vi "Create_Trajectory_Using_TrajectoryLibrary_NAT.vi"() -> ()   [LabVIEW 2019]
doc: "This utility creates trajectories based on the robot configuration, constraints and defined waypoints."
uses:
  <vilib>/Rock Robotics/WPI/ThirdParty/JAS_Junk/TrajLib/Trajectory_Library.lvlib
  <vilib>/Rock Robotics/WPI/ThirdParty/JAS_Junk/TrajLib/TypeDef/DISPLAY_WEIGHTED_WAYPOINT.ctl
  <vilib>/Rock Robotics/WPI/ThirdParty/JAS_Junk/TrajLib/TypeDef/TRAJECTORY.ctl
  <vilib>/Rock Robotics/WPI/ThirdParty/JAS_Junk/TrajLib/TypeDef/TRAJ_STATE.ctl
  <vilib>/Rock Robotics/WPI/ThirdParty/JAS_Junk/TrajLib/TypeDef/POSE2D.ctl
  <vilib>/Rock Robotics/WPI/ThirdParty/JAS_Junk/TrajLib/TypeDef/ROTATION2D.ctl
  <vilib>/Rock Robotics/WPI/ThirdParty/JAS_Junk/TrajLib/TypeDef/TRANSLATION2D.ctl
  CreateTrajectoryTypeDef/TrajCreateConfig_V3.ctl
  CreateTrajectoryENUM/TrajCreateUnitsENUM.ctl
  <vilib>/Rock Robotics/WPI/ThirdParty/JAS_Junk/TrajLib/TypeDef/TRAJ_CONSTRAINT_MECA_DRIVE_KINEMATICS.ctl
  <vilib>/Rock Robotics/WPI/ThirdParty/JAS_Junk/TrajLib/TypeDef/MECA_DRIVE_KINEMATICS.ctl
  <vilib>/Analysis/Matrix/Datatypes/RealMatrix.ctl
  <vilib>/Analysis/Matrix/NI_Matrix.lvlib
  <vilib>/Rock Robotics/WPI/ThirdParty/JAS_Junk/TrajLib/TypeDef/TRAJ_CONSTRAINT_DIIF_DRIVE_VOLTAGE.ctl
  <vilib>/Rock Robotics/WPI/ThirdParty/JAS_Junk/TrajLib/TypeDef/SIMPLE_MOTOR_FF.ctl
  <vilib>/Rock Robotics/WPI/ThirdParty/JAS_Junk/TrajLib/TypeDef/DIFF_DRIVE_KINEMATICS.ctl
  <vilib>/Rock Robotics/WPI/ThirdParty/JAS_Junk/TrajLib/TypeDef/TRAJ_CONSTRAINT_SWERVE_DRIVE_KINEMATICS.ctl
  <vilib>/Rock Robotics/WPI/ThirdParty/JAS_Junk/TrajLib/TypeDef/SWERVE_DRIVE_KINEMATICS.ctl
  <vilib>/Rock Robotics/WPI/ThirdParty/JAS_Junk/TrajLib/TypeDef/TRAJ_CONSTRAINT_CENTRIPETAL_ACCEL.ctl
  <vilib>/Utility/miscctls.llb/LVCursorListTypeDef.ctl
  <vilib>/Utility/xml.llb/Write to XML File(string).vi
  <vilib>/Utility/xml.llb/Read From XML File(string).vi
  <vilib>/Utility/inputDevices.llb/mouseAcquire.vi
  <vilib>/Rock Robotics/WPI/ThirdParty/JAS_Junk/TrajLib/TypeDef/SWERVE_DRIVE_MODULE_STATE.ctl
panel:
  out "CursIdx":i32
  out "Cursor Update Mode":i32=1
  out "Angle":dbl
  out "Scrolling":i32
  out "Index":i32
  in  "End Program":bool
  in  "Tab Control":T1(tab)
  out "Config File Read\nWithout Error":bool
  out "Config File  Read Error":errorcluster
  out "Read Config File Comment":string
  in  "Read Config File Name":path
  in  "ReadConfigFile":bool
  in  "Field Selector":string(combo)="2018 Power Up"
  in  "Units Selector":T2
  in  "MaxVelocity":dbl=50.0 format="%17.1f"
  in  "MaxAcceleration":dbl=40.0 format="%17.1f"
  out "MaxVelocity M/S":dbl=2.0 format="%17.4f"
  out "MaxAcceleration M/S^2":dbl=1.3 format="%17.4f"
  in  "Right Rear":T3={"X"=-0.5, "Y"=0.5} {"Y" format="%14.3f"; "X" format="%14.3f"}
  in  "Left Rear":T3={"X"=-0.5, "Y"=-0.5} {"Y" format="%14.3f"; "X" format="%14.3f"}
  in  "Right Front":T3={"X"=0.5, "Y"=0.5} {"Y" format="%14.3f"; "X" format="%14.3f"}
  in  "Left Front":T3={"X"=0.5, "Y"=-0.5} {"Y" format="%14.3f"; "X" format="%14.3f"}
  in  "Use Centripetal\nAcceleration\nConstaint":bool=TRUE
  out "Max Cent Accel M/S^2":dbl=1.0 format="%20.4f"
  in  "Max Cent Accel":dbl=20.0 format="%20.1f"
  in  "Use Diff Drive\nKinematic\nConstraint":bool=TRUE
  out "Wheelbase Width M":dbl=0.66 format="%20.4f"
  in  "Wheelbase Width":dbl=20.866 format="%20.1f"
  in  "Max Voltage":dbl=12.0 format="%20.4f"
  in  "SIMPLE_MOTOR_FF":T4={"Ks"=0.9, "Kv"=0.22199, "Ka"=0.04876, "KnInv"=0.0} {"KnInv" format="%13.4f"; "Ka" format="%13.4f"; "Kv" format="%13.4f"; "Ks" format="%13.4f"}
  in  "Use Diff Drive\nVoltage\nConstraint":bool=TRUE
  in  "Wheels":T3[](array[typedef])=[{"X"=0.5, "Y"=-0.5}, {"X"=0.5, "Y"=0.5}, {"X"=-0.5, "Y"=0.5}, {"X"=-0.5, "Y"=-0.5}] {"Y" format="%14.3f"; "X" format="%14.3f"}
  in  "Use Swerve Drive\nKinematics\nConstraint":bool
  in  "Use Mecanum \nDrive Kinematics\nConstraint":bool
  out "Left Front M":T3 {"Y" format="%14.3f"; "X" format="%14.3f"}
  out "Right Front M":T3 {"Y" format="%14.3f"; "X" format="%14.3f"}
  out "Left Rear M":T3 {"Y" format="%14.3f"; "X" format="%14.3f"}
  out "Right Rear M":T3 {"Y" format="%14.3f"; "X" format="%14.3f"}
  out "SIMPLE_MOTOR_FF M":T4 {"KnInv" format="%13.4f"; "Ka" format="%13.4f"; "Kv" format="%13.4f"; "Ks" format="%13.4f"}
  out "Wheels M":T3[](array[typedef]) {"Y" format="%14.3f"; "X" format="%14.3f"}
  in  "Remove Cursor":bool
  in  "Add Cursor":bool
  in  "Spline Type":enum32{"Radio Selection 1", "Radio Selection 2"}(radio)
  in  "Reverse":bool
  in  "UseWeights":bool
  in  "Calculate\nTrajectory":bool
  out "Trajectory\nCompleted\nError Free":bool
  out "Trajectory calculation error":errorcluster
  out "Position":cluster{dbl[], dbl[]}[](graph)
  out "Field Display":T5(plugin-control)
  in  "WayPoints":T6[](array[typedef])=[{"X"=15.0, "Y"=105.0, "ANGLE"=-45.0, "WEIGHT"=12.0}, {"X"=105.0, "Y"=65.0, "ANGLE"=0.0, "WEIGHT"=12.0}, {"X"=210.0, "Y"=106.0, "ANGLE"=45.0, "WEIGHT"=12.0}, {"X"=350.0, "Y"=105.0, "ANGLE"=-45.0, "WEIGHT"=12.0}] {"WEIGHT" format="%13.3f"; "ANGLE" format="%13.3f"; "Y" format="%13.3f"; "X" format="%13.3f"}
  out "Trajectory Data":cluster{dbl[], dbl[]}[](graph)
  out "differential \ndrive \nmax speed":dbl format="%15.1f"
  out "Traj States\nSize":i32
  out "Trajectory States":T7[](array[typedef]) {"POSE"."ROTATION"."SIN" format="%13.4f"; "POSE"."ROTATION"."COS" format="%13.4f"; "POSE"."ROTATION"."VALUE" format="%13.4f"; "POSE"."TRANSLATION"."Y" format="%14.3f"; "POSE"."TRANSLATION"."X" format="%14.3f"}
  in  "Trajectory JSON File Name":path
  out "JSON File Saved\nWithout Error":bool
  out "Write CSV File Error":errorcluster
  in  "PathWeaver Length Units":T10(radio)
  in  "WriteJSONFile":bool
  out "CSV File Saved\nWithout Error":bool
  in  "Trajectory Type":enum32{"Radio Selection 1", "Radio Selection 2"}(radio)
  out "Write Trajectory\nFile Error":errorcluster
  in  "Trajectory File Comment":string
  in  "Trajectory CSV File Name":path
  in  "WriteTrajFile":bool
  out "Config File Saved\nWithout Error":bool
  out "Write Config FIle Error":errorcluster
  in  "Write Config File Comment":string
  in  "Write Config File Name":path
  in  "WriteConfigFile":bool
  # "Create Trajectory  (Use LabVIEW trajectory library)"
  # "Instructions:  \n----------------\n\nThis utility will create a trajectory, show the data on the various tabs, and optionally write a \"field absolute\" or \"robot relative\" trajectory to a file. \nTo use this utility:\n\n1) Read all of these instructions!\n2) Define the robot's physical data on the \"Robot Data\" tab.  \n3) Define the robot's movement constraints on the \"Constraints\" page.  \n4) Define the trajectory on the \"Define/Create Trajectory\" tab.  These are the beginning and ending positions/headings, and internal positions/headings.  \n    Cubic splines only use the first and last \"angle\".  The other internal \"angles\" are calculated.  Quintic splines use all the defined angles.\n5) Press the \"Calculate Trajectory\".  If a good trajectory was calculated it will be displayed.  If no errors are generated the Trajectory Complete\n    light will be on.  Errors will be displayed in the error indicator.  The path can be recalculated many times before performing any other action.\n\nAfter a Trajectory has been calculated, the \"trajectory can be written to a file.  The absolute path is converted to a robot relative trajectory.  To do this:\n1) Enter a comment to be included in the file.  Anything can be entered.\n2) Select the file name.\n3) Press \"Create Trajectory File\"  If an error occurs it will be displayed in the File Creation Error indicator.\n\nNotes:\n--------\n- All the robot parameters, path, and field dimensions are in UNITS, and DEGREES.  Select UNITS from the \"Robot Data\" page.  The resulting  \n  trajectory is converted to METERS, and RADIANS to match the rest of this library!\n- The trajectory library is the same as the WPILIB spline and trajectory library for Java and C++.\n- 2019 playing field size - width: 26 ft 11.25 In = 323.25 in , length: 52 ft 5.25 in = 629.25 in  (I didn't verify this for the 2020 version.)"
  # "Read Trajectory Waypoints and Configuration from File"
  # "ROBOT DATA"
  # "UNITS/SEC"
  # "Meters/SEC"
  # "UNITS/SEC^2"
  # "Meters/SEC^2"
  # "Simulated robot max speed is: 68.266 Inches/Second"
  # "UTILITY CONFIGURATION"
  # "Diff Kinematics Constraint"
  # "Centripetal Accel Constraint"
  # "Diff Voltage Constraint"
  # "UNITS"
  # "UNITS/SEC^2"
  # "VOLTS"
  # "METERS"
  # "METERS/SEC^2"
  # "Distance is:\nUNITS"
  # "Simulated robot wheelbase is 20.87 in"
  # "Ks = Volts\nKv = VoltSec/Meter\nKa = Volt(Sec^2)/Meter"
  # "Swerve Kinematics Constraint"
  # "Mechanum Kinematics Constraint"
  # "Values\nare \nUNITS"
  # "Values\nare \nUNITS"
  # "TRAJECTORY DEFINITION"
  # "To delete array elements or the entire array, right click on the array or element, select Data Operations, then select the action to be performed."
  # "UNITS, UNITS, DEGREES, SCALAR"
  # "INCHES/SEC"
  # "Write Trajectory to File   -   CSV, and / or JSON"
  # "Write Trajectory Waypoints and Configuration to File"
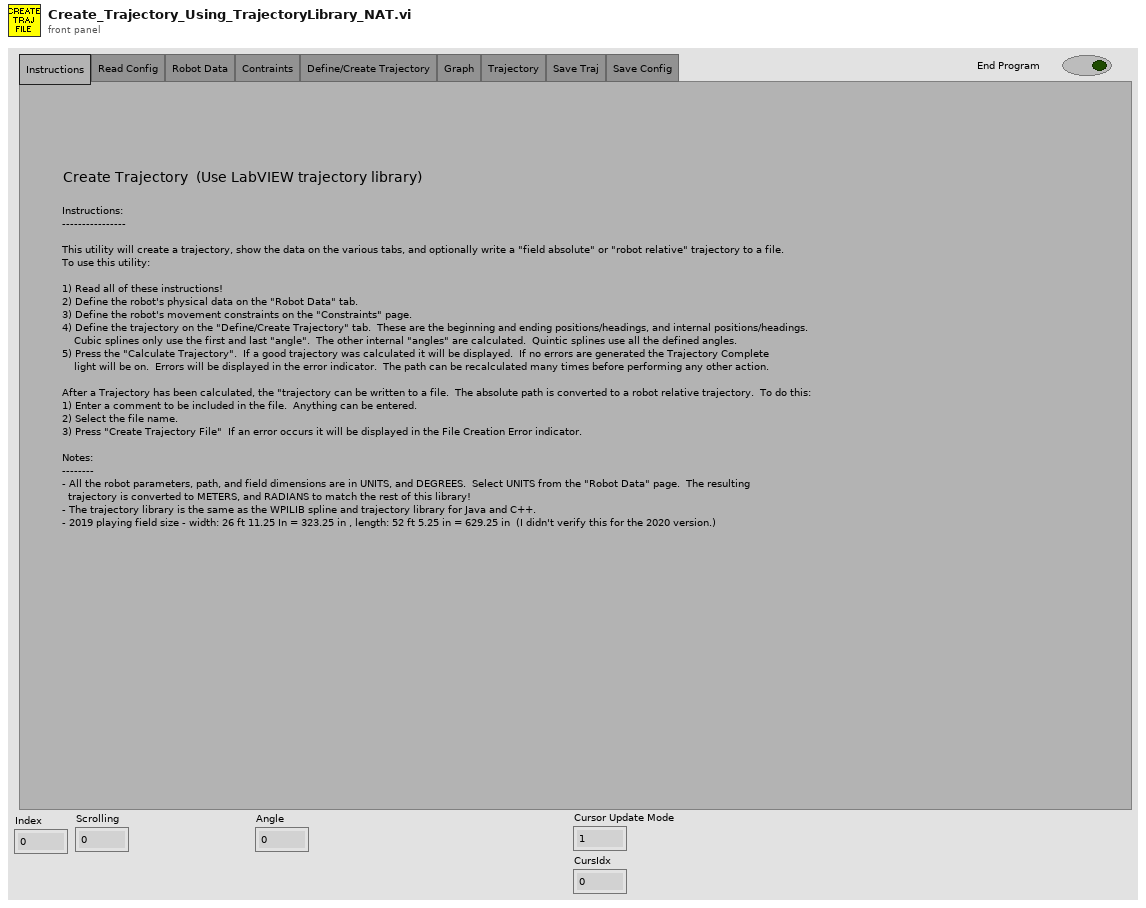
[diagram p1: front panel]
types:
  T1 = enum32{"Instructions", "Read Config", "Robot Data", "Contraints", "Define/Create Trajectory", "Graph", "Trajectory", "Save Traj", "Save Config"}
  T2 = typedef "TrajCreateUnitsENUM.ctl" = enum16{"Inches", "Feet", "Centimeters", "Meters"}
  T3 = typedef "Trajectory_Library.lvlib/TRANSLATION2D.ctl" = cluster{"X":dbl, "Y":dbl}
  T4 = typedef "Trajectory_Library.lvlib/SIMPLE_MOTOR_FF.ctl" = cluster{"Ks":dbl, "Kv":dbl, "Ka":dbl, "KnInv":dbl}
  T5 = typedef "IMAQ Image.ctl" = refnum<image>
  T6 = typedef "Trajectory_Library.lvlib/DISPLAY_WEIGHTED_WAYPOINT.ctl" = cluster{"X":dbl, "Y":dbl, "ANGLE":dbl, "WEIGHT":dbl}
  T7 = typedef "Trajectory_Library.lvlib/TRAJ_STATE.ctl" = cluster{"TimeSeconds":dbl, "Velocity":dbl, "Acceleration":dbl, "POSE":T8, "Curvature":dbl}
  T8 = typedef "Trajectory_Library.lvlib/POSE2D.ctl" = cluster{"TRANSLATION":T3, "ROTATION":T9}
  T9 = typedef "Trajectory_Library.lvlib/ROTATION2D.ctl" = cluster{"VALUE":dbl, "COS":dbl, "SIN":dbl}
  T10 = enum32{"Radio Selection 1", "Radio Selection 2", "Radio Selection 3", "Radio Selection 4", "Radio Selection 5"}
  T11 = typedef "LVCursorListTypeDef.ctl" = cluster{"Name":string, "Color":u32, "Style":u8, "Point Style":u8, "Name Visible":bool, "Allow Drag":bool, "Cursor Mode":u32, "Plot":i32, "Index":i32, "Position":cluster{"X":dbl, "Y":dbl}, "X Scale":u32, "Y Scale":u32, "Watch Plots":i32[], "Watch All Plots":bool, "Plot Area":i32, "Label Offset":cluster{"X":dbl, "Y":dbl}}[]
  T12 = typedef "Image Type" = u32
  T13 = typedef "Trajectory_Library.lvlib/TRAJECTORY.ctl" = cluster{"TotalTImeSecs":dbl, "States":T7[]}
  T14 = typedef "TrajCreateConfig_V3.ctl" = cluster{"Write Config File Name":path, "Write Config File Comment":string, "WayPoints":T6[], "TRAJECTORY_CONFIG":cluster{"MaxVelocity":dbl, "Max Acceleration":dbl, "StartVelocity":dbl, "End Velocity":dbl, "Reversed":bool, "DiffDrKineConstntDefined":bool, "CentAcellConstntDefined":bool, "DiffDrVoltConstntDefined":bool, "DIFF_DRIVE_KINE_CONSTRAINT":cluster{"Max Speed (M/S)":dbl, "DIFF_DRIVE_KINEMATICS":T15}, "CENTRIPETAL_ACCEL_CONSTRAINT":T16, "SwerveDrKineConstntDefined":bool, "SWERVE_DRIVE_KINE_CONSTRAINT":T17, "DIFF_DRIVE_VOLTAGE_CONSTRAINT":T21, "MECANUM_DRIVE_KINE_CONSTRAINT":T22, "MecanumDrKineConstntDefined":bool}, "IsCubic":bool, "Units Selector":T2, "UseWeights":bool}
  T15 = typedef "Trajectory_Library.lvlib/DIFF_DRIVE_KINEMATICS.ctl" = cluster{"TrackWidth_Meters":dbl}
  T16 = typedef "Trajectory_Library.lvlib/TRAJ_CONSTRAINT_CENTRIPETAL_ACCEL.ctl" = cluster{"Max Cent Accel":dbl}
  T17 = typedef "Trajectory_Library.lvlib/TRAJ_CONSTRAINT_SWERVE_DRIVE_KINEMATICS.ctl" = cluster{"Max Speed (M/S)":dbl, "SwerveKinematics":T18}
  T18 = typedef "Trajectory_Library.lvlib/SWERVE_DRIVE_KINEMATICS.ctl" = cluster{"NumModules":i32, "InverseKinematics":T19, "ForwardKinematics":T19, "Modules":T3[], "PrevCoR":T3, "SavedModuleStates":T20[]}
  T19 = typedef "NI_Matrix.lvlib/RealMatrix.ctl" = dbl[][]
  T20 = typedef "Trajectory_Library.lvlib/SWERVE_DRIVE_MODULE_STATE.ctl" = cluster{"Speed":dbl, "Angle":T9}
  T21 = typedef "Trajectory_Library.lvlib/TRAJ_CONSTRAINT_DIIF_DRIVE_VOLTAGE.ctl" = cluster{"Max Voltage":dbl, "DIFF_DRIVE_KINEMATICS":T15, "SIMPLE_MOTOR_FF":T4}
  T22 = typedef "Trajectory_Library.lvlib/TRAJ_CONSTRAINT_MECA_DRIVE_KINEMATICS.ctl" = cluster{"Max Speed (M/S)":dbl, "MECA_DRIVE_KINEMATICS":T23}
  T23 = typedef "Trajectory_Library.lvlib/MECA_DRIVE_KINEMATICS.ctl" = cluster{"FrontLeft":T3, "FrontRight":T3, "RearLeft":T3, "RearRight":T3, "InverseKinematics":T19, "ForwardKinematics":T19, "PrevCoR":T3}
  T24 = cluster{"Name":string, "Color":u32, "Style":u8, "Point Style":u8, "Name Visible":bool, "Allow Drag":bool, "Cursor Mode":u32, "Plot":i32, "Index":i32, "Position":cluster{"X":dbl, "Y":dbl}, "X Scale":u32, "Y Scale":u32, "Watch Plots":i32[], "Watch All Plots":bool, "Plot Area":i32, "Label Offset":cluster{"X":dbl, "Y":dbl}}
  T25 = enum8{"Enabled", "Disabled", "Disabled and Grayed Out"}
  T26 = cluster{"Horizontal":i32, "Vertical":i32, "Scrolling":i32}
  T27 = typedef "TrajectoryUtils_Field_Info.ctl" = cluster{"FIeld_File_Name":string, "Top_Left_X":i32, "Top_Left_Y":i32, "Bottom_Right_X":i32, "Bottom_Right_Y":i32, "Field_Size_X":dbl, "Field_Size_Y":dbl, "FIeld_Size_Units":string}
  T28 = typedef "TrajCreateConfig__V_Internal.ctl" = cluster{"Write Config File Name":path, "Write Config File Comment":string, "WayPoints":T6[], "TRAJECTORY_CONFIG":T29, "IsCubic":bool, "Units Selector":T2, "UseWeights":bool, "FieldName":string}
  T29 = typedef "Trajectory_Library.lvlib/TRAJ_CONFIG.ctl" = cluster{"MaxVelocity":dbl, "Max Acceleration":dbl, "StartVelocity":dbl, "End Velocity":dbl, "Reversed":bool, "Constraints":variant[]}
  T30 = typedef "Trajectory_Library.lvlib/TRAJ_CONSTRAINT_DIIF_DRIVE_KINEMATICS.ctl" = cluster{"Max Speed (M/S)":dbl, "DIFF_DRIVE_KINEMATICS":T15, "Max Accel (M/S2)":dbl}
  T31 = typedef "Trajectory_Library.lvlib/TRAJ_CONSTRAINT_DIIF_DRIVE_VOLTAGE.ctl" = cluster{"Max Voltage":dbl, "DIFF_DRIVE_KINEMATICS":T15, "SIMPLE_MOTOR_FF":T32}
  T32 = typedef "Trajectory_Library.lvlib/SIMPLE_MOTOR_FF.ctl" = cluster{"Ks":dbl, "Kv":dbl, "Ka":dbl}
  T33 = typedef "Trajectory_Library.lvlib/TRAJ_CONSTRAINT_SWERVE_DRIVE_KINEMATICS.ctl" = cluster{"Max Speed (M/S)":dbl, "SwerveKinematics":T34}
  T34 = typedef "Trajectory_Library.lvlib/SWERVE_DRIVE_KINEMATICS.ctl" = cluster{"NumModules":i32, "InverseKinematics":T19, "ForwardKinematics":T19, "Modules":T3[], "PrevCoR":T3}
  T35 = typedef "Trajectory_Library.lvlib/WEIGHTED_WAYPOINT.ctl" = cluster{"TRANSLATION":T3, "ROTATION":T9, "SCALAR":dbl}
  T36 = typedef "Trajectory_Library.lvlib/SPLINE_CTRL_VECTOR.ctl" = cluster{"Xs":dbl[], "Ys":dbl[]}
  T37 = typedef "Trajectory_Library.lvlib/CHASSIS_SPEEDS.ctl" = cluster{"vX":dbl, "vY":dbl, "vOmega":dbl}
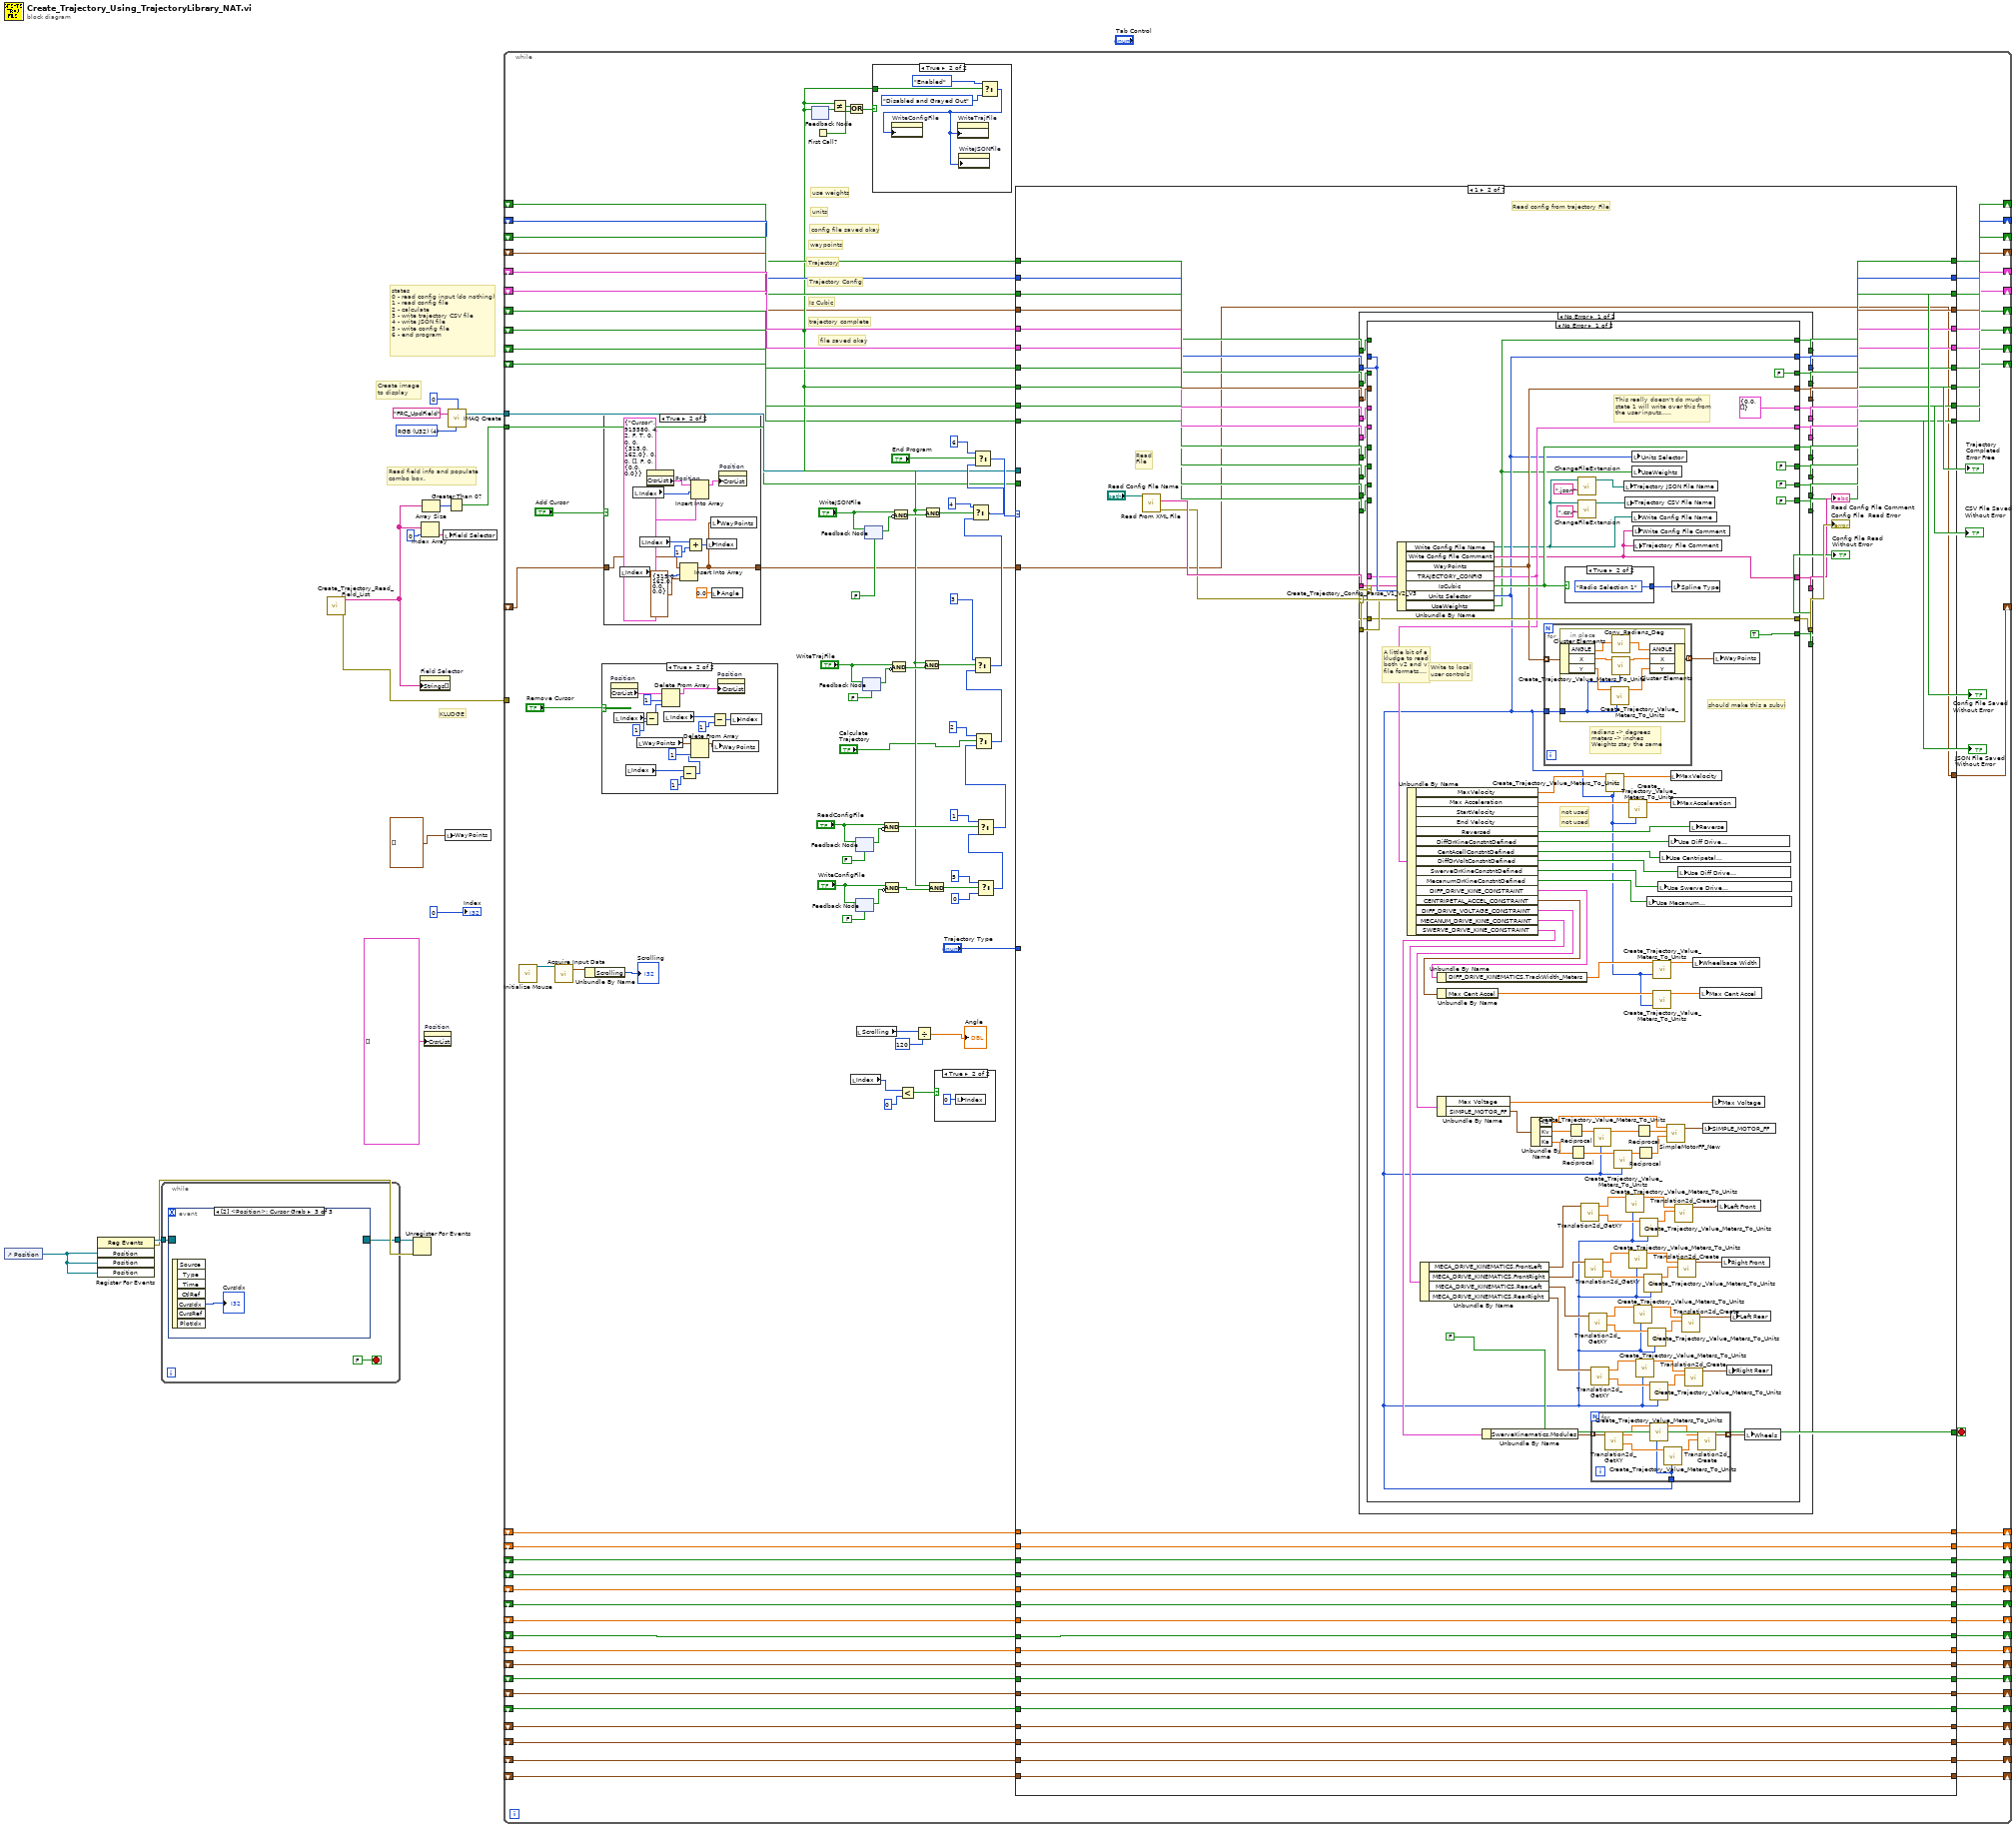
[diagram p0: block diagram]
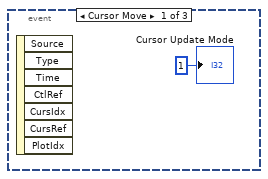
[diagram p2: hidden frame]
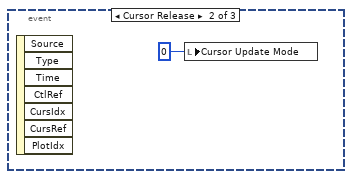
[diagram p3: hidden frame]
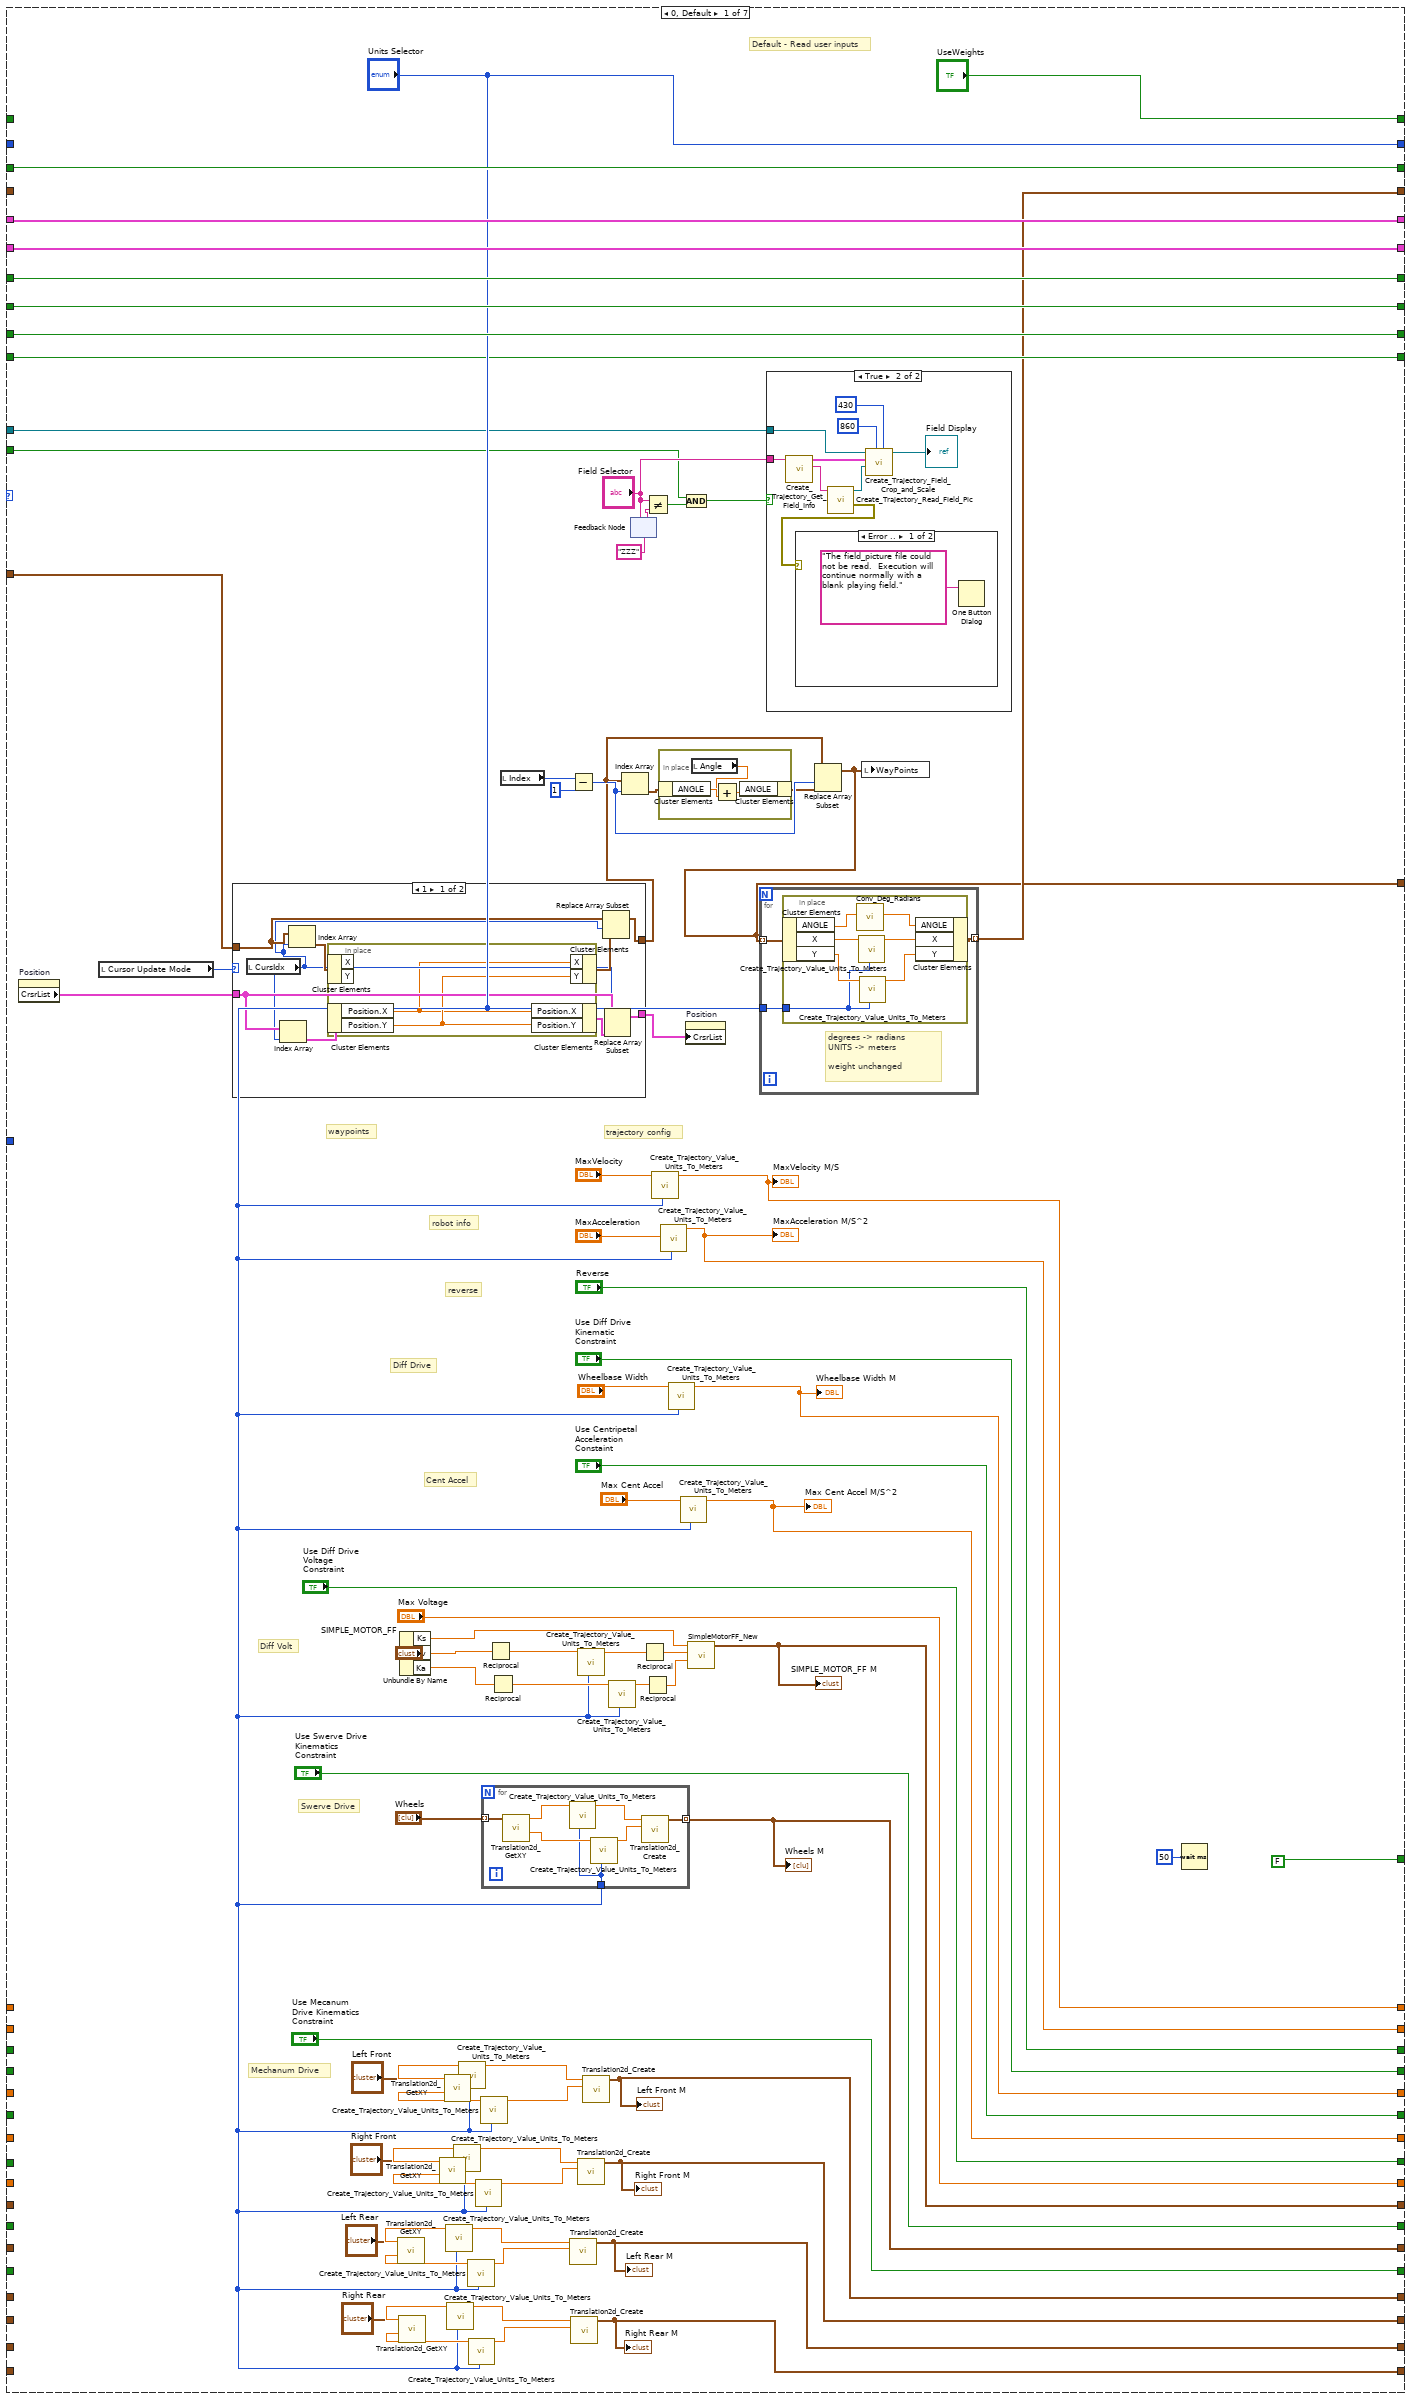
[diagram p4: hidden frame]
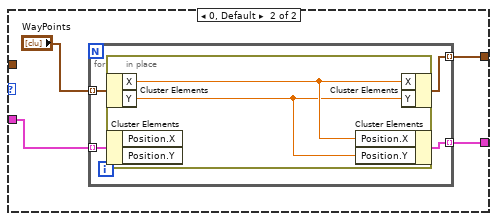
[diagram p5: hidden frame]
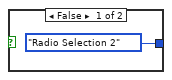
[diagram p8: hidden frame]
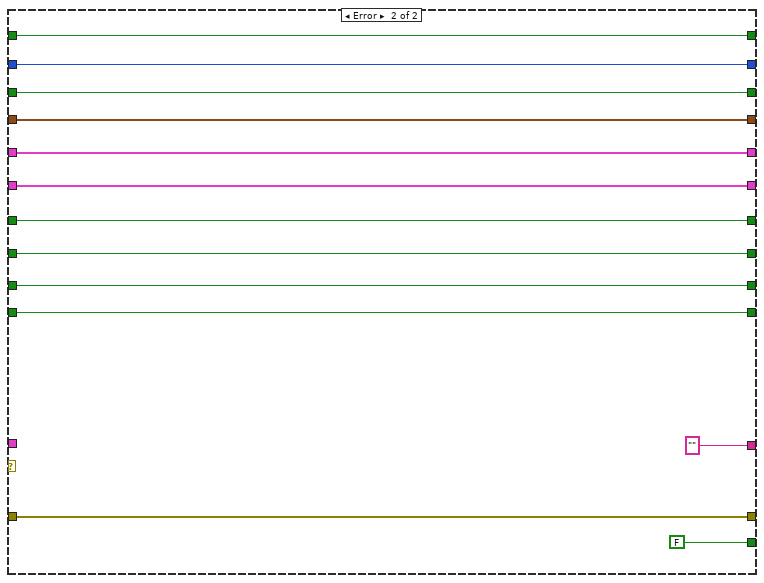
[diagram p9: hidden frame]
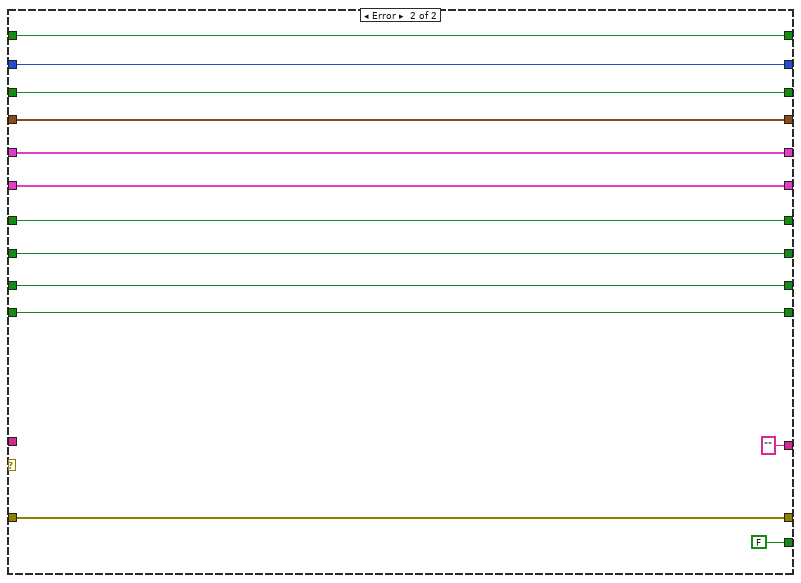
[diagram p10: hidden frame]
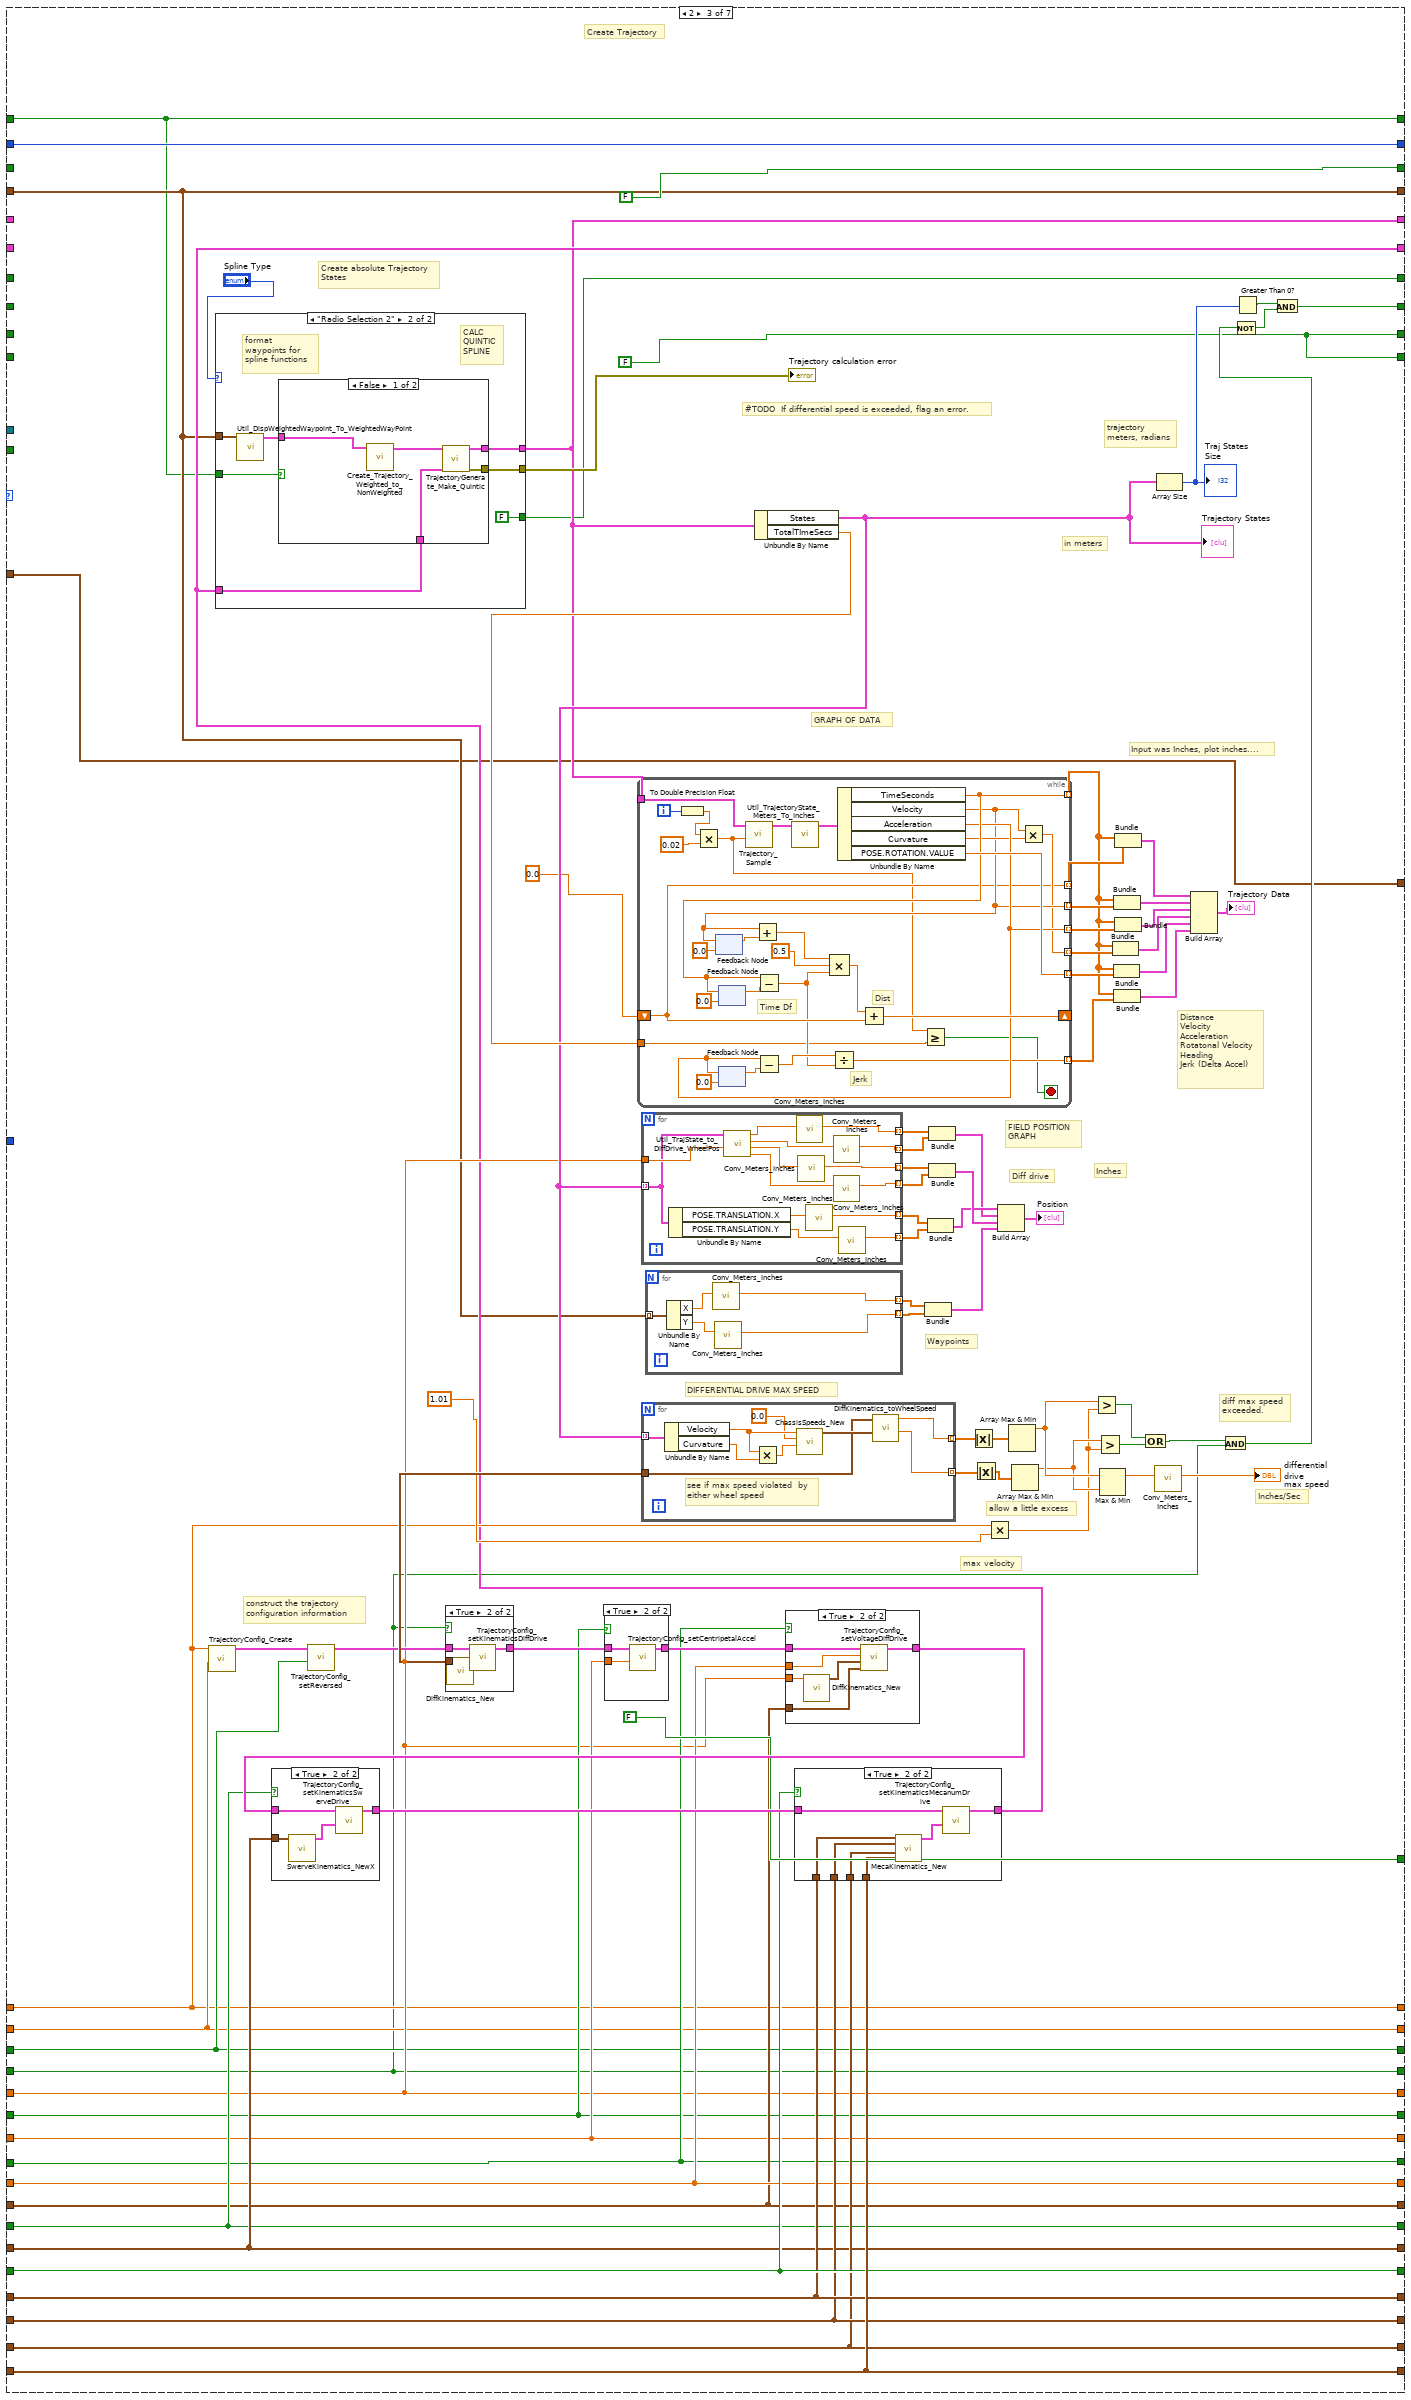
[diagram p11: hidden frame]
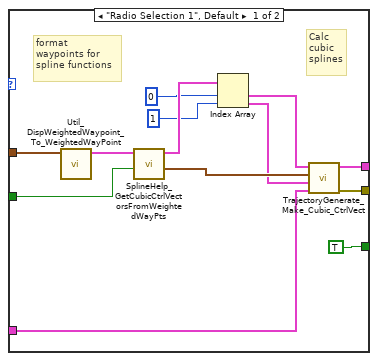
[diagram p13: hidden frame]
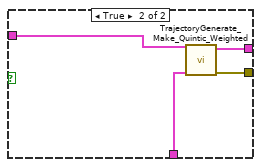
[diagram p14: hidden frame]
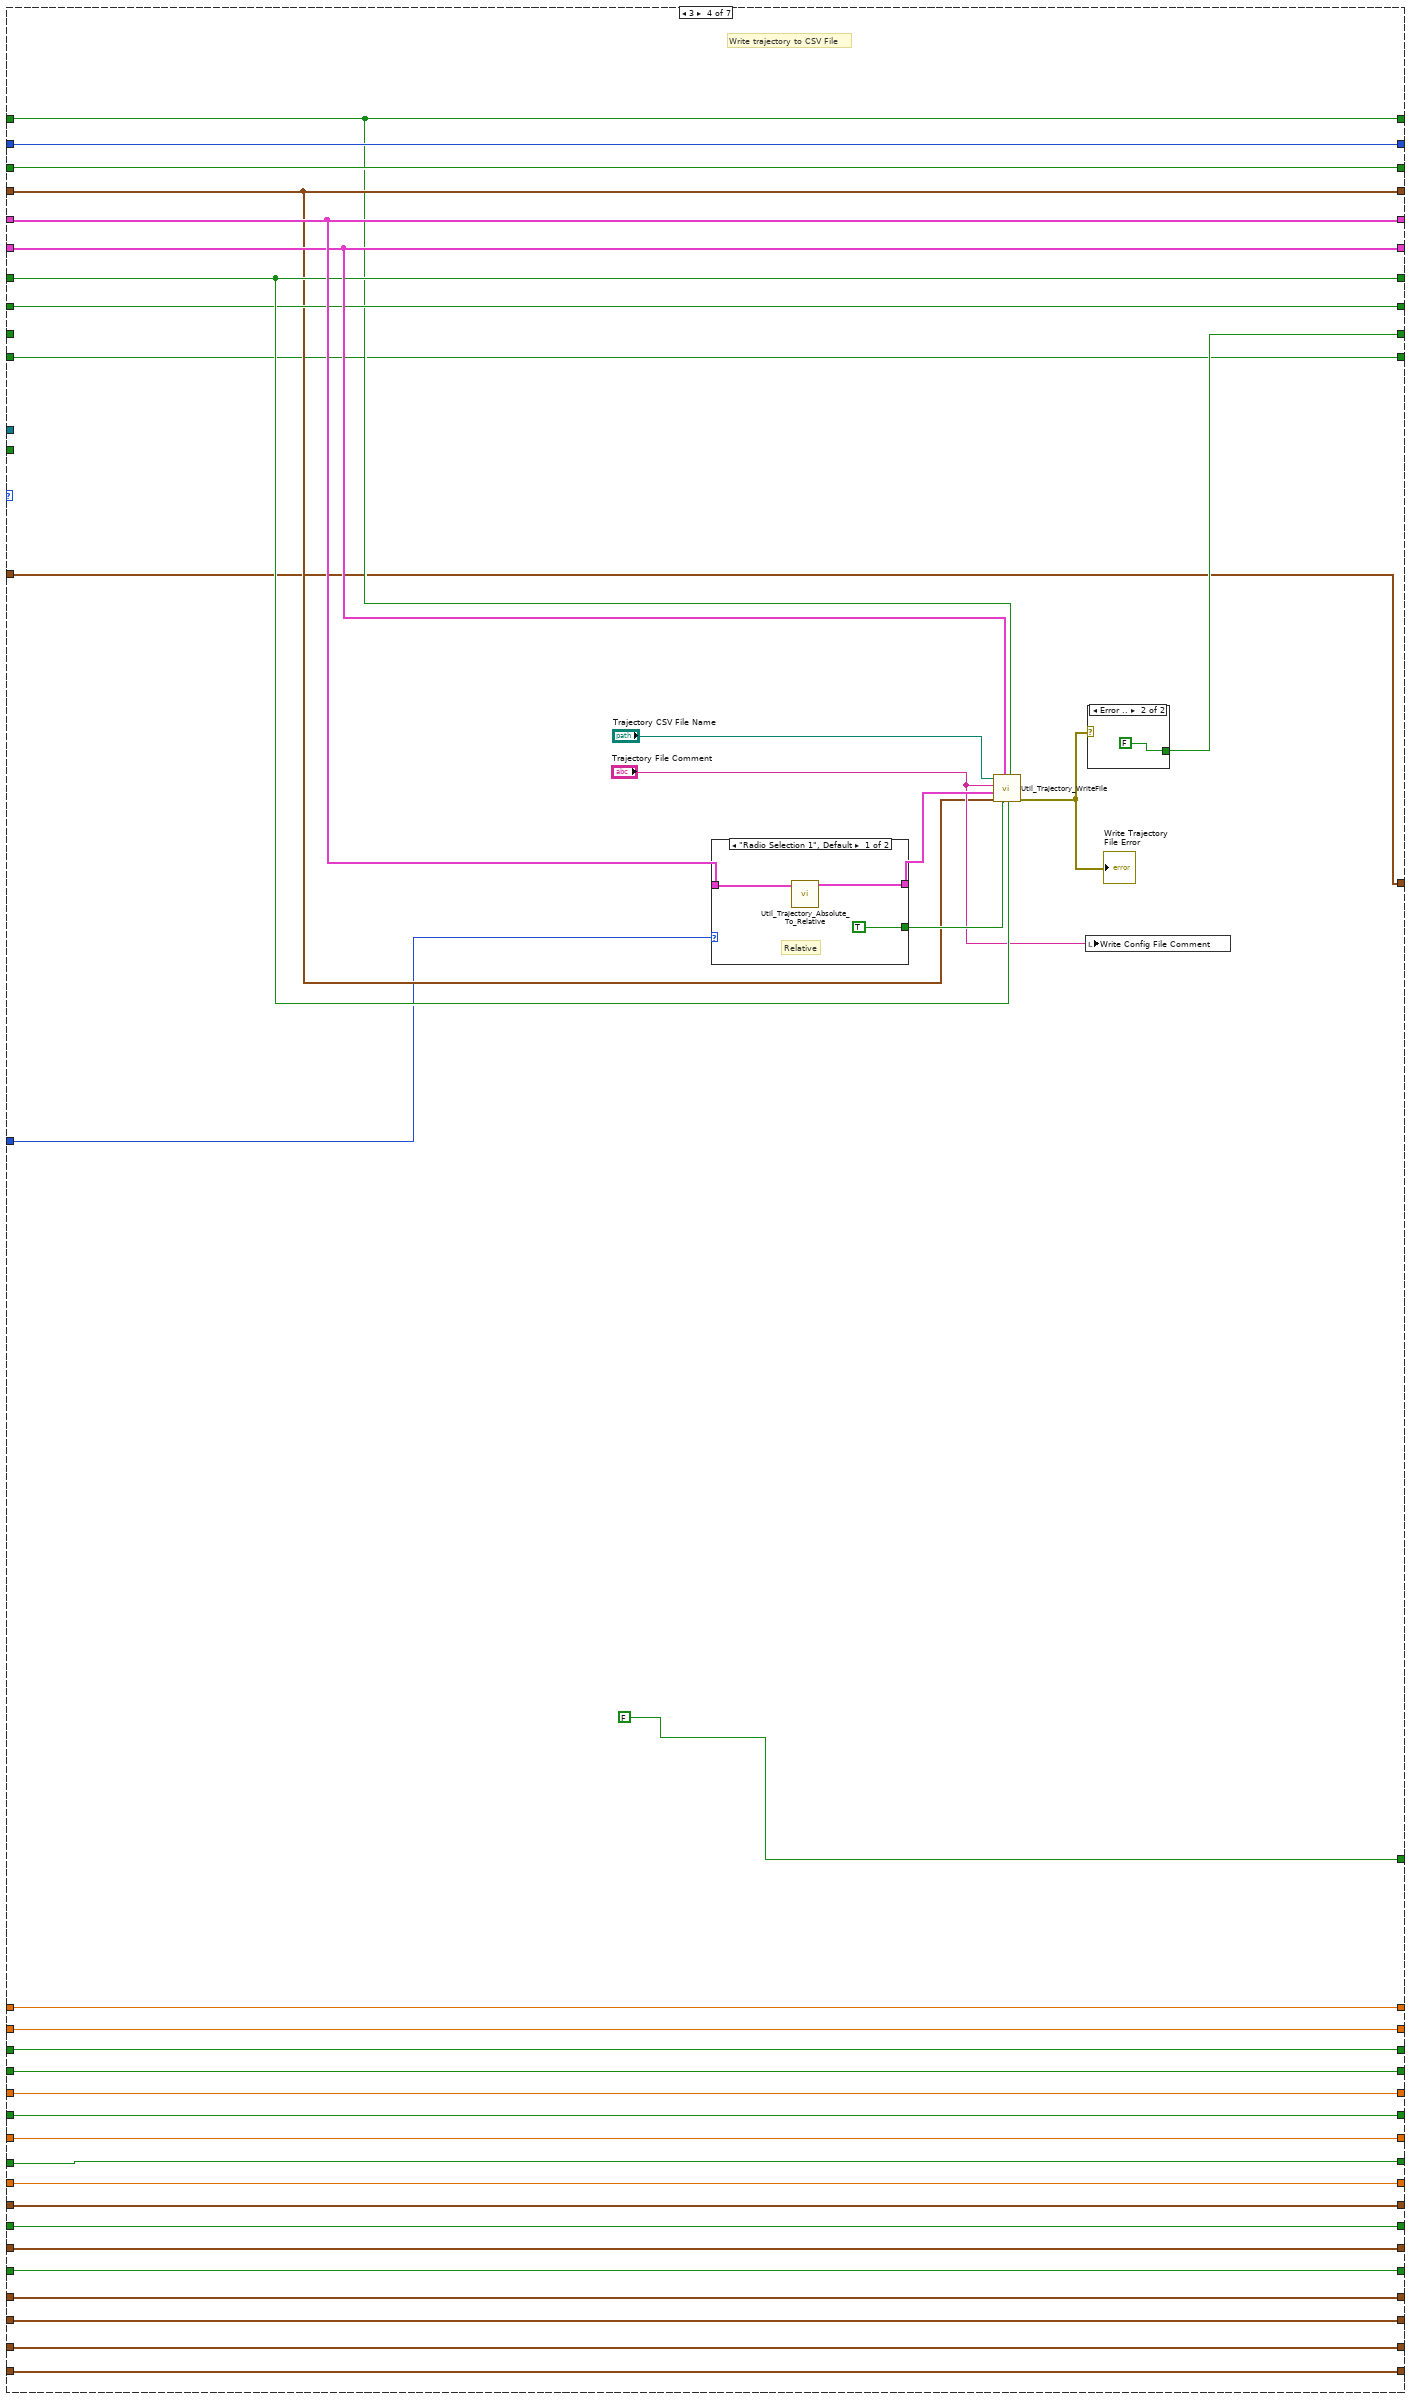
[diagram p19: hidden frame]
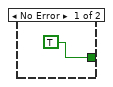
[diagram p20: hidden frame]
diagram:
  w12 = T12 4 items=["Grayscale (U8)", "Grayscale (I16)", "Grayscale (SGL)", "Complex (CSG)", "RGB (U32)", "HSL (U32)", "RGB (U64)", "Grayscale (U16)"] ("Image Type")
  # "Create image \nto display"
  # "KLUDGE"
  # "Read field info and populate\ncombo box."
  # "states\n0 - read config input (do nothing)\n1 - read config file\n2 - calculate\n3 - write trajectory CSV file\n4 - write JSON file\n5 - write config file\n6 - end program"
  n1 = control-ref of="Position"() -> (w4:refnum<vi>)
  n2 = register-events(w4, w4, w4) -> (reference out=w3:refnum<event-registration>, error out=w1:errorcluster)  [unwired: 2 in]
  n3 = while {
    tunnel: w3 -> [w20]
    tunnel: [w19] -> w2
    stop <- FALSE stop-if-true
    n4 = event shown="[2] <Position>: Cursor Grab" {
      selector: w20 -> [_ _ _]
      dyn-events: [_ _ _] -> w19
      timeout: _ -> [_ _ _]
      event Cursor Move {
        n5 = event-data() -> ()  [unwired: 1 in, 7 out]
        "Cursor Update Mode" <- 1
      }
      event Cursor Release {
        n6 = event-data() -> ()  [unwired: 1 in, 7 out]
        n7 = local write "Cursor Update Mode"(0 ("Wapoint Update Mode")) -> ()
      }
      event Cursor Grab {
        n8 = event-data() -> ("CursIdx"=→"CursIdx":i32)  [unwired: 1 in, 6 out]
      }
    }
  }
  n9 = call "Create_Trajectory_Read_Field_List.vi"() -> ("error out"=w15:errorcluster, "section names"=w10:string[])  [unwired: 10 in]
  n10 = Unregister For Events(event registration refnum=w2, error in=w1) -> ()  [unwired: 1 out]
  n11 = property on="Field Selector" class="CmbBox"("Strings[]"=w10) -> ()  [unwired: 2 in, 2 out]
  n12 = Index Array(array=w10, index=0) -> (element=w16:string)
  n13 = Array Size(array=w10) -> (size(s)=w9:i32)
  n14 = property on="Position" class="XYGraph (strict)"("CrsrList"=T11 [] ("Cursor List")) -> ()  [unwired: 2 in, 2 out]
  n15 = local write "Field Selector"(w16) -> ()
  n16 = local write "WayPoints"(T6[] [] ("WayPoints")) -> ()
  n17 = Greater Than 0?(x=w9) -> (x > 0?=w8:bool)
  n18 = call "IMAQ Create"("Border Size"=0, "Image Name"="FRC_UpdField", "Image Type"=w12) -> ("New Image"=w11:T5)  [unwired: 2 in, 1 out]
  n19 = while {
    shift-right: [w127] -> _
    shift-left: _ -> [w126]
    shift-right: [w125] -> _
    shift-left: _ -> [w124]
    shift-right: [w111] -> _
    shift-left: _ -> [w112]
    shift-right: [w113] -> _
    shift-left: _ -> [w29]
    shift-right: [w110] -> _
    shift-left: _ -> [w50]
    shift-right: [w106] -> _
    shift-left: _ -> [w107]
    shift-right: [w96] -> _
    shift-left: _ -> [w101]
    shift-right: [w105] -> _
    shift-left: _ -> [w100]
    shift-right: [w97] -> _
    shift-left: _ -> [w104]
    shift-right: [w98] -> _
    shift-left: _ -> [w103]
    shift-right: [w99] -> _
    shift-left: _ -> [w102]
    shift-right: [w95] -> _
    shift-left: _ -> [w93]
    shift-right: [w94] -> _
    shift-left: _ -> [w92]
    shift-right: [w89] -> _
    shift-left: _ -> [w90]
    shift-right: [w88] -> _
    shift-left: _ -> [w91]
    shift-right: [w86] -> _
    shift-left: _ -> [w87]
    shift-right: [w82] -> _
    shift-left: _ -> [w84]
    shift-right: [w83] -> _
    shift-left: _ -> [w85]
    shift-right: [w79] -> _
    shift-left: _ -> [w81]
    shift-right: [w78] -> _
    shift-left: _ -> [w80]
    shift-right: [w72] -> _
    shift-left: _ -> [w75]
    shift-right: [w73] -> _
    shift-left: _ -> [w76]
    shift-right: [w74] -> _
    shift-left: _ -> [w77]
    shift-right: [w60] -> _
    shift-left: _ -> [w59]
    shift-right: [w58] -> _
    shift-left: _ -> [w57]
    shift-right: [w56] -> _
    shift-left: _ -> [w55]
    shift-right: [w45] -> _
    shift-left: _ -> [w44]
    tunnel: w15 -> [_]
    tunnel: w11 -> [w42]
    tunnel: w8 -> [w41]
    shift-right: [w28] -> _
    shift-left: _ -> [w27]
    stop <- w108 stop-if-true
    # "use weights"
    # "units"
    # "config file saved okay"
    # "file saved okay"
    # "trajectory complete"
    # "Is Cubic"
    # "waypoints"
    # "Trajectory Config"
    # "Trajectory"
    n20 = call <vilib>:"Initialize Mouse.vi"() -> ("device ID"=w33:refnum<k1>)  [unwired: 10 in, 1 out]
    n21 = call-poly <vilib>:"Acquire Input Data.vi"("device ID"=w33) -> ("axis info"=w34:T26)  [unwired: 15 in, 3 out]
    n22 = Unbundle By Name(w34) -> ("Scrolling"=→"Scrolling":i32)
    n23 = case shown="True" "Remove Cursor" {
      frame False {
      }
      frame True {
        n24 = property on="Position" class="XYGraph (strict)"() -> ("CrsrList"=w922:T11)  [unwired: 2 in, 2 out]
        n25 = local read "Index"() -> (w913:i32)
        n26 = local read "Index"() -> (w908:i32)
        n27 = local read "WayPoints"() -> (w915:T6[])
        n28 = Subtract(x=w913, y=1) -> (x-y=w911:i32)
        n29 = Delete From Array(array=w922, length=1, index=w911) -> (array with subset deleted=w920:T11)  [unwired: 1 out]
        n30 = local read "Index"() -> (w919:i32)
        n31 = Subtract(x=w908, y=1) -> (x-y=w909:i32)
        n32 = Delete From Array(array=w915, length=1, index=w909) -> (array with subset deleted=w916:T6[])  [unwired: 1 out]
        n33 = Subtract(x=w919, y=1) -> (x-y=w917:i32)
        n34 = local write "WayPoints"(w916) -> ()
        n35 = property on="Position" class="XYGraph (strict)"("CrsrList"=w920) -> ()  [unwired: 2 in, 2 out]
        n36 = local write "Index"(w917) -> ()
      }
    }
    n37 = case shown="True" "Add Cursor" {
      tunnel: [w923 w925] -> w30
      tunnel: w27 -> [w923 w924]
      frame False {
      }
      frame True {
        n38 = local read "Index"() -> (w929:i32)
        n39 = local read "Index"() -> (w934:i32)
        n40 = local read "Index"() -> (w931:i32)
        n41 = property on="Position" class="XYGraph (strict)"() -> ("CrsrList"=w935:T11)  [unwired: 2 in, 2 out]
        n42 = Insert Into Array(array=w924, index=w929, new element=T6 {"X"=315.0, "Y"=162.0, "ANGLE"=0.0, "WEIGHT"=0.0} ("new element/subarray")) -> (w925:T6[])
        n43 = Add(x=w931, y=1) -> (x+y=w933:i32)
        n44 = Insert Into Array(array=w935, index=w934, new element=T24 {"Name"="Cursor", "Color"=915580, "Style"=4, "Point Style"=2, "Name Visible"=FALSE, "Allow Drag"=TRUE, "Cursor Mode"=0, "Plot"=0, "Index"=0, "Position"={"X"=315.0, "Y"=162.0}, "X Scale"=0, "Y Scale"=0, "Watch Plots"=[], "Watch All Plots"=FALSE, "Plot Area"=0, "Label Offset"={"X"=0.0, "Y"=0.0}} ("new element/subarray")) -> (w930:T11)
        n45 = local write "Index"(w933) -> ()
        n46 = local write "WayPoints"(w925) -> ()
        n47 = local write "Angle"(0.0 ("Angle")) -> ()
        n48 = property on="Position" class="XYGraph (strict)"("CrsrList"=w930) -> ()  [unwired: 2 in, 2 out]
      }
    }
    n49 = feedback #1() -> (w64:bool)  [unwired: 1 in]
    n50 = feedback-in #1(w50) -> ()
    n51 = First Call?() -> (First Call?: T/F=w62:bool)
    n52 = Not Equal?(x=w50, y=w64) -> (x != y?=w63:bool)
    n53 = Or(x=w63, y=w62) -> (x .or. y?=w61:bool)
    n54 = local read "Index"() -> (w40:i32)
    n55 = feedback #2(FALSE ("CreateCmdList")) -> (w130:bool)
    n56 = feedback-in #2("ReadConfigFile") -> ()
    n57 = feedback #3(FALSE ("CreateCmdList")) -> (w71:bool)
    n58 = feedback-in #3("WriteConfigFile") -> ()
    n59 = local read "Scrolling"() -> (w32:i32)
    n60 = feedback #4(FALSE ("CreateCmdList")) -> (w132:bool)
    n61 = feedback-in #4("WriteTrajFile") -> ()
    n62 = feedback #5(FALSE ("CreateCmdList")) -> (w54:bool)
    n63 = feedback-in #5("WriteJSONFile") -> ()
    n64 = case shown="True" w61 {
      tunnel: w50 -> [_ w940]
      frame False {
      }
      frame True {
        n65 = Select(t=T25."Enabled" ("Disabled"), s=w940, f=T25."Disabled and Grayed Out" ("Disabled")) -> (s? t:f=w937:T25)
        n66 = property on="WriteConfigFile" class="Bool"("DisabledEnum"=w937) -> ()  [unwired: 2 in, 2 out]
        n67 = property on="WriteTrajFile" class="Bool"("DisabledEnum"=w937) -> ()  [unwired: 2 in, 2 out]
        n68 = property on="WriteJSONFile" class="Bool"("DisabledEnum"=w937) -> ()  [unwired: 2 in, 2 out]
      }
    }
    n69 = Compound Arithmetic op=AND("ReadConfigFile", invert w130) -> (w115:bool)
    n70 = Compound Arithmetic op=AND("WriteConfigFile", invert w71) -> (w24:bool)
    n71 = Compound Arithmetic op=AND("WriteTrajFile", invert w132) -> (w109:bool)
    n72 = Compound Arithmetic op=AND("WriteJSONFile", invert w54) -> (w51:bool)
    n73 = Less?(x=w40, y=0) -> (x < y?=w38:bool)
    n74 = Divide(x=w32, y=120) -> (x/y=→"Angle":dbl)
    n75 = And(x=w50, y=w109) -> (x .and. y?=w120:bool)
    n76 = And(x=w50, y=w51) -> (x .and. y?=w48:bool)
    n77 = And(x=w50, y=w24) -> (x .and. y?=w65:bool)
    n78 = case shown="True" w38 {
      frame False {
      }
      frame True {
        n79 = local write "Index"(0 ("index")) -> ()
      }
    }
    n80 = Select(t=5, s=w65, f=0) -> (s? t:f=w67:i32)
    n81 = Select(t=1, s=w115, f=w67) -> (s? t:f=w116:i32)
    n82 = Select(t=2, s="Calculate\nTrajectory", f=w116) -> (s? t:f=w118:i32)
    n83 = Select(t=3, s=w120, f=w118) -> (s? t:f=w47:i32)
    n84 = Select(t=4, s=w48, f=w47) -> (s? t:f=w46:i32)
    n85 = Select(t=6, s="End Program", f=w46) -> (s? t:f=w114:i32)
    n86 = case shown="1" w114 {
      tunnel: w81 -> [_ w306 w496 w672 w722 w861 w896]
      tunnel: w85 -> [_ w304 w498 w674 w724 w863 w894]
      tunnel: w80 -> [_ w307 w487 w671 w721 w860 w897]
      tunnel: w84 -> [_ w305 w497 w673 w723 w862 w895]
      tunnel: w87 -> [_ w303 w499 w675 w725 w864 w893]
      tunnel: w91 -> [_ w301 w500 w677 w727 w866 w891]
      tunnel: w90 -> [_ w302 w501 w676 w726 w865 w892]
      tunnel: w92 -> [_ w300 w502 w678 w728 w867 w890]
      tunnel: w93 -> [_ w299 w503 w679 w729 w868 w889]
      tunnel: w102 -> [_ w298 w507 w680 w730 w869 w888]
      tunnel: w103 -> [_ w297 w506 w681 w731 w870 w887]
      tunnel: w104 -> [_ w296 w505 w682 w732 w871 w886]
      tunnel: w100 -> [_ w294 w508 w684 w734 w873 w884]
      tunnel: [w215 w284 w491 w689 w738 w875 w905] -> w127
      tunnel: w126 -> [w215 w290 _ w689 w738 w875 w905]
      tunnel: [w214 w283 w492 w688 w737 w855 w904] -> w125
      tunnel: w124 -> [w214 w289 _ w688 w737 w855 w904]
      tunnel: [w213 w282 w490 w687 w736 w854 w903] -> w111
      tunnel: [w145 w285 w484 w664 w715 w856 w906] -> w113
      tunnel: w29 -> [_ w291 w484 w664 w715 w856 w906]
      tunnel: w112 -> [w213 w288 _ w687 w736 w854 w903]
      tunnel: [w212 w281 w515 w686 w735 w874 w902] -> w110
      tunnel: w50 -> [w212 w287 _ w686 w735 w874 w902]
      tunnel: [FALSE FALSE FALSE FALSE FALSE FALSE TRUE] -> w108
      tunnel: [w209 w280 w478 w685 w712 w853 w901] -> w106
      tunnel: w107 -> [w209 w286 _ _ w712 w853 w901]
      tunnel: [w169 w294 w508 w684 w734 w873 w884] -> w105
      tunnel: w101 -> [_ w295 w504 w683 w733 w872 w885]
      tunnel: ["Use Mecanum \nDrive Kinematics\nConstraint" w298 w507 w680 w730 w869 w888] -> w99
      tunnel: [w190 w297 w506 w681 w731 w870 w887] -> w98
      tunnel: [w171 w296 w505 w682 w732 w871 w886] -> w97
      tunnel: [w170 w295 w504 w683 w733 w872 w885] -> w96
      tunnel: [w156 w299 w503 w679 w729 w868 w889] -> w95
      tunnel: ["Use Swerve Drive\nKinematics\nConstraint" w300 w502 w678 w728 w867 w890] -> w94
      tunnel: ["Max Voltage" w302 w501 w676 w726 w865 w892] -> w89
      tunnel: [w168 w301 w500 w677 w727 w866 w891] -> w88
      tunnel: ["Use Diff Drive\nVoltage\nConstraint" w303 w499 w675 w725 w864 w893] -> w86
      tunnel: [w201 w304 w498 w674 w724 w863 w894] -> w83
      tunnel: ["Use Centripetal\nAcceleration\nConstaint" w305 w497 w673 w723 w862 w895] -> w82
      tunnel: [w198 w306 w496 w672 w722 w861 w896] -> w79
      tunnel: ["Use Diff Drive\nKinematic\nConstraint" w307 w487 w671 w721 w860 w897] -> w78
      tunnel: w77 -> [_ w308 w495 w670 w720 w859 w898]
      tunnel: w76 -> [_ w309 w494 w669 w719 w858 w899]
      tunnel: w75 -> [_ w310 w493 w668 w718 w857 w900]
      tunnel: ["Reverse" w308 w495 w670 w720 w859 w898] -> w74
      tunnel: [w195 w309 w494 w669 w719 w858 w899] -> w73
      tunnel: [w194 w310 w493 w668 w718 w857 w900] -> w72
      tunnel: [w193 w275 FALSE ("File Saved\nWithout\nError") w667 w717 w847 w883] -> w60
      tunnel: w59 -> [w193 w274 _ w667 w717 _ w883]
      tunnel: ["Units Selector" w272 w485 w666 w716 w845 w882] -> w58
      tunnel: w57 -> [_ w273 w485 w666 w716 w845 w882]
      tunnel: ["UseWeights" w271 w479 w663 w714 w843 w881] -> w56
      tunnel: w55 -> [_ w270 w479 w663 w714 w843 w881]
      tunnel: [w153 w269 w478 w662 w713 w842 w880] -> w45
      tunnel: w44 -> [w153 w268 _ w662 _ w842 w880]
      tunnel: "Trajectory Type" -> [_ _ _ w661 w711 _ _]
      tunnel: w42 -> [w149 _ _ _ _ _ _]
      tunnel: w41 -> [w146 _ _ _ _ _ _]
      tunnel: w30 -> [w135 w267 w462 w660 w702 w841 w879]
      tunnel: [w138 w267 w462 w660 w702 w841 w879] -> w28
      frame 0, Default {
        # "reverse"
        # "robot info"
        # "Diff Drive"
        # "Cent Accel"
        # "Diff Volt"
        # "Swerve Drive"
        # "Mechanum Drive"
        # "trajectory config"
        # "waypoints"
        # "Default - Read user inputs"
        n87 = property on="Position" class="XYGraph (strict)"() -> ("CrsrList"=w137:T11)  [unwired: 2 in, 2 out]
        n88 = local read "Cursor Update Mode"() -> (w136:i32)
        n89 = case shown="1" w136 {
          tunnel: w137 -> [w221 w233]
          tunnel: w135 -> [w225 _]
          tunnel: [w223 w231] -> w134
          tunnel: [w219 w230] -> w144
          frame 1 {
            n90 = local read "CursIdx"() -> (w220:i32)
            n91 = Index Array(array=w221, index=w220) -> (element=w227:T24)
            n92 = Index Array(array=w225, index=w220) -> (element=w226:T6)
            n93 = in-place {
              n94 = in-place-cluster #6(w226) -> ()  [unwired: 2 out]
              n95 = in-place-cluster #7(w227) -> ("Position.X"=w228:dbl, "Position.Y"=w229:dbl)
              n96 = in-place-cluster #7("Position.X"=w228, "Position.Y"=w229) -> (w222:T24)
              n97 = in-place-cluster #6("X"=w228, "Y"=w229) -> (w224:T6)
            }
            n98 = Replace Array Subset(array=w225, new element=w224, index=w220) -> (w223:T6[])
            n99 = Replace Array Subset(array=w221, new element=w222, index=w220) -> (w219:T11)
          }
          frame 0, Default {
            n100 = for {
              tunnel: w233 -> [w237] mode=indexing
              tunnel: "WayPoints" -> [w236] mode=indexing
              tunnel: [w235] -> w231 mode=indexing
              tunnel: [w234] -> w230 mode=indexing
              n101 = in-place {
                n102 = in-place-cluster #8(w236) -> ("X"=w239:dbl, "Y"=w238:dbl)
                n103 = in-place-cluster #9(w237) -> ()  [unwired: 2 out]
                n104 = in-place-cluster #9("Position.X"=w239, "Position.Y"=w238) -> (w234:T24)
                n105 = in-place-cluster #8("X"=w239, "Y"=w238) -> (w235:T6)
              }
            }
          }
        }
        n106 = call <vilib>:"Translation2d_GetXY.vi"("In Translation"="Left Rear") -> ("Y"=w179:dbl, "X"=w181:dbl)  [unwired: 9 in]
        n107 = call <vilib>:"Translation2d_GetXY.vi"("In Translation"="Right Rear") -> ("Y"=w174:dbl, "X"=w176:dbl)  [unwired: 9 in]
        n108 = Unbundle By Name("SIMPLE_MOTOR_FF") -> ("Ks"=w166:dbl, "Kv"=w165:dbl, "Ka"=w158:dbl)
        n109 = call <vilib>:"Translation2d_GetXY.vi"("In Translation"="Right Front") -> ("Y"=w184:dbl, "X"=w186:dbl)  [unwired: 9 in]
        n110 = call <vilib>:"Translation2d_GetXY.vi"("In Translation"="Left Front") -> ("Y"=w189:dbl, "X"=w192:dbl)  [unwired: 9 in]
        n111 = call "Create_Trajectory_Value_Units_To_Meters.vi"("Units Selector"="Units Selector", "Units"=w181) -> ("Meters"=w180:dbl)  [unwired: 9 in]
        n112 = call "Create_Trajectory_Value_Units_To_Meters.vi"("Units Selector"="Units Selector", "Units"=w176) -> ("Meters"=w175:dbl)  [unwired: 9 in]
        n113 = call "Create_Trajectory_Value_Units_To_Meters.vi"("Units Selector"="Units Selector", "Units"=w186) -> ("Meters"=w185:dbl)  [unwired: 9 in]
        n114 = call "Create_Trajectory_Value_Units_To_Meters.vi"("Units Selector"="Units Selector", "Units"=w192) -> ("Meters"=w191:dbl)  [unwired: 9 in]
        n115 = call "Create_Trajectory_Value_Units_To_Meters.vi"("Units Selector"="Units Selector", "Units"=w179) -> ("Meters"=w178:dbl)  [unwired: 9 in]
        n116 = call "Create_Trajectory_Value_Units_To_Meters.vi"("Units Selector"="Units Selector", "Units"=w174) -> ("Meters"=w173:dbl)  [unwired: 9 in]
        n117 = call "Create_Trajectory_Value_Units_To_Meters.vi"("Units Selector"="Units Selector", "Units"=w184) -> ("Meters"=w183:dbl)  [unwired: 9 in]
        n118 = call "Create_Trajectory_Value_Units_To_Meters.vi"("Units Selector"="Units Selector", "Units"=w189) -> ("Meters"=w188:dbl)  [unwired: 9 in]
        n119 = for {
          tunnel: "Wheels" -> [w252] mode=indexing
          tunnel: [w251] -> w156 mode=indexing
          tunnel: "Units Selector" -> [w250]
          n120 = call <vilib>:"Translation2d_GetXY.vi"("In Translation"=w252) -> ("Y"=w254:dbl, "X"=w256:dbl)  [unwired: 9 in]
          n121 = call "Create_Trajectory_Value_Units_To_Meters.vi"("Units Selector"=w250, "Units"=w256) -> ("Meters"=w255:dbl)  [unwired: 9 in]
          n122 = call "Create_Trajectory_Value_Units_To_Meters.vi"("Units Selector"=w250, "Units"=w254) -> ("Meters"=w253:dbl)  [unwired: 9 in]
          n123 = call <vilib>:"Translation2d_Create.vi"("Y"=w253, "X"=w255) -> ("TRANSLATION"=w251:T3)  [unwired: 9 in]
        }
        "Wheels M" <- w156
        n124 = Reciprocal(x=w165) -> (1/x=w164:dbl)
        n125 = Reciprocal(x=w158) -> (1/x=w161:dbl)
        n126 = local read "Index"() -> (w142:i32)
        n127 = Subtract(x=w142, y=1) -> (x-y=w143:i32)
        n128 = call <vilib>:"Translation2d_Create.vi"("Y"=w178, "X"=w180) -> ("TRANSLATION"=w170:T3)  [unwired: 9 in]
        "Left Rear M" <- w170
        n129 = call <vilib>:"Translation2d_Create.vi"("Y"=w173, "X"=w175) -> ("TRANSLATION"=w169:T3)  [unwired: 9 in]
        "Right Rear M" <- w169
        n130 = call "Create_Trajectory_Value_Units_To_Meters.vi"("Units Selector"="Units Selector", "Units"=w164) -> ("Meters"=w163:dbl)  [unwired: 9 in]
        n131 = call <vilib>:"Translation2d_Create.vi"("Y"=w183, "X"=w185) -> ("TRANSLATION"=w171:T3)  [unwired: 9 in]
        "Right Front M" <- w171
        n132 = call <vilib>:"Translation2d_Create.vi"("Y"=w188, "X"=w191) -> ("TRANSLATION"=w190:T3)  [unwired: 9 in]
        "Left Front M" <- w190
        n133 = call "Create_Trajectory_Value_Units_To_Meters.vi"("Units Selector"="Units Selector", "Units"=w161) -> ("Meters"=w160:dbl)  [unwired: 9 in]
        n134 = Index Array(array=w134, index=w143) -> (element=w139:T6)
        n135 = feedback #10("ZZZ" ("Field Selector")) -> (w152:string)
        n136 = feedback-in #10("Field Selector") -> ()
        n137 = Reciprocal(x=w163) -> (1/x=w162:dbl)
        n138 = Reciprocal(x=w160) -> (1/x=w159:dbl)
        n139 = Not Equal?(x="Field Selector", y=w152) -> (x != y?=w148:bool)
        n140 = call "Create_Trajectory_Value_Units_To_Meters.vi"("Units Selector"="Units Selector", "Units"="MaxVelocity") -> ("Meters"=w194:dbl)  [unwired: 9 in]
        "MaxVelocity M/S" <- w194
        n141 = in-place {
          n142 = in-place-cluster #11(w139) -> ("ANGLE"=w218:dbl)
          n143 = local read "Angle"() -> (w217:dbl)
          n144 = Add(x=w217, y=w218) -> (x+y=w216:dbl)
          n145 = in-place-cluster #11("ANGLE"=w216) -> (w141:T6)
        }
        n146 = call "Create_Trajectory_Value_Units_To_Meters.vi"("Units Selector"="Units Selector", "Units"="MaxAcceleration") -> ("Meters"=w195:dbl)  [unwired: 9 in]
        "MaxAcceleration M/S^2" <- w195
        n147 = call "Create_Trajectory_Value_Units_To_Meters.vi"("Units Selector"="Units Selector", "Units"="Wheelbase Width") -> ("Meters"=w198:dbl)  [unwired: 9 in]
        "Wheelbase Width M" <- w198
        n148 = call "Create_Trajectory_Value_Units_To_Meters.vi"("Units Selector"="Units Selector", "Units"="Max Cent Accel") -> ("Meters"=w201:dbl)  [unwired: 9 in]
        "Max Cent Accel M/S^2" <- w201
        n149 = And(x=w146, y=w148) -> (x .and. y?=w147:bool)
        n150 = property on="Position" class="XYGraph (strict)"("CrsrList"=w144) -> ()  [unwired: 2 in, 2 out]
        n151 = call <vilib>:"SimpleMotorFF_New.vi"("Ka"=w159, "Kv"=w162, "Ks"=w166) -> ("SIMPLE_MOTOR_FF"=w168:T4)  [unwired: 8 in]
        "SIMPLE_MOTOR_FF M" <- w168
        n152 = case shown="True" w147 {
          tunnel: "Field Selector" -> [_ w264]
          tunnel: w149 -> [_ w263]
          frame False {
          }
          frame True {
            n153 = call "Create_Trajectory_Get_Field_Info.vi"("Field Selector"=w264) -> ("File"=w265:string, "input cluster"=w262:T27)  [unwired: 9 in]
            n154 = call "Create_Trajectory_Read_Field_Pic.vi"("file name"=w265) -> ("Image Error"=w257:errorcluster, "Image Data"=w261:T5)  [unwired: 7 in, 2 out]
            n155 = case shown="Error .." w257 {
              frame Error {
                n156 = One Button Dialog(message="The field_picture file could not be read.  Execution will continue normally with a blank playing field.") -> ()  [unwired: 1 in, 1 out]
              }
              frame No Error {
              }
            }
            n157 = call "Create_Trajectory_Field_Crop_and_Scale.vi"("Disp Y Size Pixel"=430, "Disp X Size Pixel"=860, "Field Image"=w261, "field Info"=w262, "Display Image"=w263) -> ("Disp Image Out"=→"Field Display":T5)  [unwired: 5 in, 1 out]
          }
        }
        n158 = Replace Array Subset(array=w134, new element=w141, index=w143) -> (w138:T6[])
        n159 = for {
          tunnel: w138 -> [w242] mode=indexing
          tunnel: [w241] -> w145 mode=indexing
          tunnel: "Units Selector" -> [w240]
          # "degrees -> radians\nUNITS -> meters\n\nweight unchanged"
          n160 = in-place {
            in-place-border: w240 -> [w243]
            n161 = in-place-cluster #12(w242) -> ("ANGLE"=w244:dbl, "X"=w249:dbl, "Y"=w247:dbl)
            n162 = call <vilib>:"Conv_Deg_Radians.vi"("Degress"=w244) -> ("Radians"=w245:dbl)  [unwired: 10 in]
            n163 = call "Create_Trajectory_Value_Units_To_Meters.vi"("Units Selector"=w243, "Units"=w249) -> ("Meters"=w248:dbl)  [unwired: 9 in]
            n164 = call "Create_Trajectory_Value_Units_To_Meters.vi"("Units Selector"=w243, "Units"=w247) -> ("Meters"=w246:dbl)  [unwired: 9 in]
            n165 = in-place-cluster #12("ANGLE"=w245, "X"=w248, "Y"=w246) -> (w241:T6)
          }
        }
        n166 = local write "WayPoints"(w138) -> ()
        n167 = Wait (ms)(milliseconds to wait=u32 50) -> ()  [unwired: 1 out]
      }
      frame 1 {
        # "Read\nFile"
        # "Read config from trajectory File"
        n168 = call-poly <vilib>:"Read From XML File.vi"("XML File Path"="Read Config File Name") -> ("error out"=w279:errorcluster, "XML Elements"=w292:string)  [unwired: 8 in, 1 out]
        n169 = case shown="No Error" w279 {
          tunnel: w292 -> [w318 _]
          tunnel: w291 -> [w338 w461]
          tunnel: w290 -> [w337 w460]
          tunnel: w289 -> [w336 w459]
          tunnel: w288 -> [w335 w458]
          tunnel: w287 -> [w334 w457]
          tunnel: w286 -> [w333 w456]
          tunnel: [w332 w461] -> w285
          tunnel: [w331 w460] -> w284
          tunnel: [w330 w459] -> w283
          tunnel: [w329 w458] -> w282
          tunnel: [w328 w457] -> w281
          tunnel: [w327 w456] -> w280
          tunnel: w279 -> [w317 w455]
          tunnel: [w325 w455] -> w278
          tunnel: [w324 FALSE] -> w277
          tunnel: [w326 "" ("Write Config File Comment")] -> w276
          tunnel: [w323 w452] -> w275
          tunnel: w274 -> [w322 w452]
          tunnel: w273 -> [w319 w451]
          tunnel: [w321 w451] -> w272
          tunnel: [w315 w450] -> w271
          tunnel: w270 -> [w314 w450]
          tunnel: [w313 w449] -> w269
          tunnel: w268 -> [w312 w449]
          frame No Error {
            # "parse\nXML"
            # "A little bit of a \nkludge to read \nboth v2 and v1\nfile formats...."
            n170 = call "Create_Trajectory_Config_Parse_V1_V2_V3.vi"("error in (no error)"=w317, "Units Selector"=w319, "XML Elements"=w318) -> ("error out"=w320:errorcluster, "TrajCreateConfig"=w316:T28)  [unwired: 7 in]
            n171 = case shown="No Error" w320 {
              tunnel: w338 -> [_ w448]
              tunnel: w337 -> [_ w447]
              tunnel: w336 -> [_ w446]
              tunnel: w335 -> [_ w445]
              tunnel: w334 -> [_ w444]
              tunnel: w333 -> [_ w443]
              tunnel: [w409 w448] -> w332
              tunnel: [T13 {"TotalTImeSecs"=0.0, "States"=[]} ("TRAJECTORY") w447] -> w331
              tunnel: [w408 w446] -> w330
              tunnel: [w410 w445] -> w329
              tunnel: [FALSE w444] -> w328
              tunnel: [FALSE ("File Saved\nWithout\nError") w443] -> w327
              tunnel: w316 -> [w415 _]
              tunnel: [w387 "" ("Write Config File Comment")] -> w326
              tunnel: w320 -> [w413 w441]
              tunnel: [w413 w441] -> w325
              tunnel: [TRUE FALSE] -> w324
              tunnel: [FALSE ("File Saved\nWithout\nError") w439] -> w323
              tunnel: w322 -> [_ w439]
              tunnel: w319 -> [_ w438]
              tunnel: [w346 w438] -> w321
              tunnel: [w343 w437] -> w315
              tunnel: w314 -> [_ w437]
              tunnel: [FALSE ("File Saved\nWithout\nError") w436] -> w313
              tunnel: w312 -> [_ w436]
              frame No Error {
                # "This really doesn't do much\nstate 1 will write over this from\nthe user inputs....."
                # "Write to local\nuser controls"
                # "not used"
                # "not used"
                # "should make this a subvi"
                n172 = Unbundle By Name(w415) -> ("Write Config File Name"=w340:path, "Write Config File Comment"=w387:string, "WayPoints"=w409:T6[], "TRAJECTORY_CONFIG"=w408:T29, "IsCubic"=w410:bool, "Units Selector"=w346:T2, "UseWeights"=w343:bool)
                n173 = Unbundle By Name(w408) -> ("MaxVelocity"=w405:dbl, "Max Acceleration"=w404:dbl, "Reversed"=w403:bool, "DiffDrKineConstntDefined"=w402:bool, "CentAcellConstntDefined"=w401:bool, "DiffDrVoltConstntDefined"=w400:bool, "SwerveDrKineConstntDefined"=w399:bool, "MecanumDrKineConstntDefined"=w398:bool, "DIFF_DRIVE_KINE_CONSTRAINT"=w397:T30, "CENTRIPETAL_ACCEL_CONSTRAINT"=w394:T16, "DIFF_DRIVE_VOLTAGE_CONSTRAINT"=w391:T31, "MECANUM_DRIVE_KINE_CONSTRAINT"=w389:T22, "SWERVE_DRIVE_KINE_CONSTRAINT"=w388:T33)  [unwired: 2 out]
                n174 = Unbundle By Name(w389) -> ("MECA_DRIVE_KINEMATICS.FrontLeft"=w362:T3, "MECA_DRIVE_KINEMATICS.FrontRight"=w363:T3, "MECA_DRIVE_KINEMATICS.RearLeft"=w364:T3, "MECA_DRIVE_KINEMATICS.RearRight"=w365:T3)
                n175 = Unbundle By Name(w397) -> ("DIFF_DRIVE_KINEMATICS.TrackWidth_Meters"=w395:dbl)
                n176 = Unbundle By Name(w394) -> ("Max Cent Accel"=w392:dbl)
                n177 = Unbundle By Name(w391) -> ("Max Voltage"=w390:dbl, "SIMPLE_MOTOR_FF"=w348:T32)
                n178 = Unbundle By Name(w388) -> ("SwerveKinematics.Modules"=w382:T3[])
                n179 = Unbundle By Name(w348) -> ("Ks"=w357:dbl, "Kv"=w356:dbl, "Ka"=w349:dbl)
                n180 = for {
                  tunnel: w409 -> [w426] mode=indexing
                  tunnel: [w425] -> w345 mode=indexing
                  tunnel: w346 -> [w424]
                  # "radians -> degrees\nmeters -> inches\nWeights stay the same"
                  n181 = in-place {
                    in-place-border: w424 -> [w427]
                    n182 = in-place-cluster #13(w426) -> ("ANGLE"=w428:dbl, "X"=w433:dbl, "Y"=w431:dbl)
                    n183 = call "Create_Trajectory_Value_Meters_To_Units.vi"("Units Selector"=w427, "Meters"=w431) -> ("Units"=w430:dbl)  [unwired: 9 in]
                    n184 = call <vilib>:"Conv_Radians_Deg.vi"("Radians"=w428) -> ("Degrees"=w429:dbl)  [unwired: 10 in]
                    n185 = call "Create_Trajectory_Value_Meters_To_Units.vi"("Units Selector"=w427, "Meters"=w433) -> ("Units"=w432:dbl)  [unwired: 9 in]
                    n186 = in-place-cluster #13("ANGLE"=w429, "X"=w432, "Y"=w430) -> (w425:T6)
                  }
                }
                n187 = case shown="True" w410 {
                  tunnel: [enum32{"Radio Selection 1", "Radio Selection 2"}."Radio Selection 2" ("Spline Type") enum32{"Radio Selection 1", "Radio Selection 2"}."Radio Selection 1" ("Spline Type")] -> w411
                  frame False {
                  }
                  frame True {
                  }
                }
                n188 = Reciprocal(x=w356) -> (1/x=w355:dbl)
                n189 = Reciprocal(x=w349) -> (1/x=w352:dbl)
                n190 = call "ChangeFileExtension.vi"("NewExtenion"=".json", "In FileName"=w340) -> ("Out FileName"=w339:path)  [unwired: 9 in]
                n191 = call "ChangeFileExtension.vi"("NewExtenion"=".csv", "In FileName"=w340) -> ("Out FileName"=w386:path)  [unwired: 9 in]
                n192 = call <vilib>:"Translation2d_GetXY.vi"("In Translation"=w362) -> ("Y"=w379:dbl, "X"=w381:dbl)  [unwired: 9 in]
                n193 = call <vilib>:"Translation2d_GetXY.vi"("In Translation"=w363) -> ("Y"=w375:dbl, "X"=w377:dbl)  [unwired: 9 in]
                n194 = call <vilib>:"Translation2d_GetXY.vi"("In Translation"=w364) -> ("Y"=w371:dbl, "X"=w373:dbl)  [unwired: 9 in]
                n195 = for {
                  tunnel: w382 -> [w419] mode=indexing
                  tunnel: [w418] -> w383 mode=indexing
                  tunnel: w346 -> [w417]
                  n196 = call <vilib>:"Translation2d_GetXY.vi"("In Translation"=w419) -> ("Y"=w421:dbl, "X"=w423:dbl)  [unwired: 9 in]
                  n197 = call "Create_Trajectory_Value_Meters_To_Units.vi"("Units Selector"=w417, "Meters"=w423) -> ("Units"=w422:dbl)  [unwired: 9 in]
                  n198 = call "Create_Trajectory_Value_Meters_To_Units.vi"("Units Selector"=w417, "Meters"=w421) -> ("Units"=w420:dbl)  [unwired: 9 in]
                  n199 = call <vilib>:"Translation2d_Create.vi"("Y"=w420, "X"=w422) -> ("TRANSLATION"=w418:T3)  [unwired: 9 in]
                }
                n200 = call <vilib>:"Translation2d_GetXY.vi"("In Translation"=w365) -> ("Y"=w367:dbl, "X"=w369:dbl)  [unwired: 9 in]
                n201 = call "Create_Trajectory_Value_Meters_To_Units.vi"("Units Selector"=w346, "Meters"=w355) -> ("Units"=w354:dbl)  [unwired: 9 in]
                n202 = call "Create_Trajectory_Value_Meters_To_Units.vi"("Units Selector"=w346, "Meters"=w405) -> ("Units"=w406:dbl)  [unwired: 9 in]
                n203 = call "Create_Trajectory_Value_Meters_To_Units.vi"("Units Selector"=w346, "Meters"=w352) -> ("Units"=w351:dbl)  [unwired: 9 in]
                n204 = local write "Trajectory JSON File Name"(w339) -> ()
                n205 = local write "Trajectory CSV File Name"(w386) -> ()
                n206 = call "Create_Trajectory_Value_Meters_To_Units.vi"("Units Selector"=w346, "Meters"=w381) -> ("Units"=w380:dbl)  [unwired: 9 in]
                n207 = call "Create_Trajectory_Value_Meters_To_Units.vi"("Units Selector"=w346, "Meters"=w404) -> ("Units"=w407:dbl)  [unwired: 9 in]
                n208 = call "Create_Trajectory_Value_Meters_To_Units.vi"("Units Selector"=w346, "Meters"=w377) -> ("Units"=w376:dbl)  [unwired: 9 in]
                n209 = local write "Units Selector"(w346) -> ()
                n210 = local write "UseWeights"(w343) -> ()
                n211 = local write "Write Config File Name"(w340) -> ()
                n212 = local write "Write Config File Comment"(w387) -> ()
                n213 = local write "Trajectory File Comment"(w387) -> ()
                n214 = call "Create_Trajectory_Value_Meters_To_Units.vi"("Units Selector"=w346, "Meters"=w373) -> ("Units"=w372:dbl)  [unwired: 9 in]
                n215 = Reciprocal(x=w354) -> (1/x=w353:dbl)
                n216 = call "Create_Trajectory_Value_Meters_To_Units.vi"("Units Selector"=w346, "Meters"=w369) -> ("Units"=w368:dbl)  [unwired: 9 in]
                n217 = Reciprocal(x=w351) -> (1/x=w350:dbl)
                n218 = call "Create_Trajectory_Value_Meters_To_Units.vi"("Units Selector"=w346, "Meters"=w379) -> ("Units"=w378:dbl)  [unwired: 9 in]
                n219 = call "Create_Trajectory_Value_Meters_To_Units.vi"("Units Selector"=w346, "Meters"=w375) -> ("Units"=w374:dbl)  [unwired: 9 in]
                n220 = local write "Use Mecanum \nDrive Kinematics\nConstraint"(w398) -> ()
                n221 = call "Create_Trajectory_Value_Meters_To_Units.vi"("Units Selector"=w346, "Meters"=w371) -> ("Units"=w370:dbl)  [unwired: 9 in]
                n222 = call "Create_Trajectory_Value_Meters_To_Units.vi"("Units Selector"=w346, "Meters"=w367) -> ("Units"=w366:dbl)  [unwired: 9 in]
                n223 = call "Create_Trajectory_Value_Meters_To_Units.vi"("Units Selector"=w346, "Meters"=w395) -> ("Units"=w396:dbl)  [unwired: 9 in]
                n224 = call "Create_Trajectory_Value_Meters_To_Units.vi"("Units Selector"=w346, "Meters"=w392) -> ("Units"=w393:dbl)  [unwired: 9 in]
                n225 = local write "Use Swerve Drive\nKinematics\nConstraint"(w399) -> ()
                n226 = local write "Use Centripetal\nAcceleration\nConstaint"(w401) -> ()
                n227 = call <vilib>:"SimpleMotorFF_New.vi"("Ka"=w350, "Kv"=w353, "Ks"=w357) -> ("SIMPLE_MOTOR_FF"=w347:T4)  [unwired: 8 in]
                n228 = local write "Use Diff Drive\nKinematic\nConstraint"(w402) -> ()
                n229 = local write "MaxVelocity"(w406) -> ()
                n230 = local write "MaxAcceleration"(w407) -> ()
                n231 = local write "Spline Type"(w411) -> ()
                n232 = call <vilib>:"Translation2d_Create.vi"("Y"=w378, "X"=w380) -> ("TRANSLATION"=w361:T3)  [unwired: 9 in]
                n233 = local write "Use Diff Drive\nVoltage\nConstraint"(w400) -> ()
                n234 = call <vilib>:"Translation2d_Create.vi"("Y"=w374, "X"=w376) -> ("TRANSLATION"=w360:T3)  [unwired: 9 in]
                n235 = call <vilib>:"Translation2d_Create.vi"("Y"=w370, "X"=w372) -> ("TRANSLATION"=w359:T3)  [unwired: 9 in]
                n236 = call <vilib>:"Translation2d_Create.vi"("Y"=w366, "X"=w368) -> ("TRANSLATION"=w358:T3)  [unwired: 9 in]
                n237 = local write "Reverse"(w403) -> ()
                n238 = local write "Wheelbase Width"(w396) -> ()
                n239 = local write "Max Cent Accel"(w393) -> ()
                n240 = local write "SIMPLE_MOTOR_FF"(w347) -> ()
                n241 = local write "Max Voltage"(w390) -> ()
                n242 = local write "WayPoints"(w345) -> ()
                n243 = local write "Left Front"(w361) -> ()
                n244 = local write "Right Front"(w360) -> ()
                n245 = local write "Right Rear"(w358) -> ()
                n246 = local write "Left Rear"(w359) -> ()
                n247 = local write "Wheels"(w383) -> ()
              }
              frame Error {
              }
            }
          }
          frame Error {
          }
        }
        "Config File Read\nWithout Error" <- w277
        "Config File  Read Error" <- w278
        "Read Config File Comment" <- w276
      }
      frame 2 {
        w478 = FALSE ("File Saved\nWithout\nError")
        # "Input was Inches, plot inches...."
        # "Distance\nVelocity\nAcceleration\nRotatonal Velocity\nHeading\nJerk (Delta Accel)"
        # "#TODO  If differential speed is exceeded, flag an error."
        # "Waypoints"
        # "diff max speed\nexceeded."
        # "Inches/Sec"
        # "Inches"
        # "max velocity"
        # "Create Trajectory"
        # "allow a little excess"
        # "in meters"
        # "Diff drive"
        # "FIELD POSITION\nGRAPH"
        # "GRAPH OF DATA"
        # "construct the trajectory\nconfiguration information"
        # "trajectory \nmeters, radians"
        # "DIFFERENTIAL DRIVE MAX SPEED"
        # "Create absolute Trajectory\nStates"
        n248 = call <vilib>:"TrajectoryConfig_Create.vi"("MaxAcceleration"=w494, "MaxVelocity"=w493) -> ("TRAJECTORY_CONFIG"=w510:T29)  [unwired: 9 in]
        n249 = call <vilib>:"TrajectoryConfig_setReversed.vi"("Reversed"=w495, "inTRAJECTORY_CONFIG"=w510) -> ("outTRAJECTORY_CONFIG"=w509:T29)  [unwired: 9 in]
        n250 = call <vilib>:"DiffKinematics_New.vi"("TrackWidth_Meters"=w496) -> ("DIFF_DRIVE_KINEMATICS"=w523:T15)  [unwired: 10 in]
        n251 = case shown="True" w487 {
          tunnel: w509 -> [w647 w650]
          tunnel: [w647 w649] -> w536
          tunnel: w523 -> [_ w648]
          frame False {
          }
          frame True {
            n252 = call <vilib>:"TrajectoryConfig_setKinematicsDiffDrive.vi"("DIFF_DRIVE_KINEMATICS"=w648, "inTRAJECTORY_CONFIG"=w650) -> ("outTRAJECTORY_CONFIG"=w649:T29)  [unwired: 9 in]
          }
        }
        n253 = case shown="True" w497 {
          tunnel: w536 -> [w643 w646]
          tunnel: w498 -> [_ w645]
          tunnel: [w643 w644] -> w528
          frame False {
          }
          frame True {
            n254 = call <vilib>:"TrajectoryConfig_setCentripetalAccel.vi"("Max Cent Accel"=w645, "inTRAJECTORY_CONFIG"=w646) -> ("outTRAJECTORY_CONFIG"=w644:T29)  [unwired: 9 in]
          }
        }
        n255 = for {
          tunnel: w484 -> [w613] mode=indexing
          tunnel: [w610] -> w483 mode=indexing
          tunnel: [w609] -> w482 mode=indexing
          n256 = Unbundle By Name(w613) -> ("X"=w612:dbl, "Y"=w611:dbl)
          n257 = call <vilib>:"Conv_Meters_Inches.vi"("Meters"=w612) -> ("Inches"=w610:dbl)  [unwired: 10 in]
          n258 = call <vilib>:"Conv_Meters_Inches.vi"("Meters"=w611) -> ("Inches"=w609:dbl)  [unwired: 10 in]
        }
        n259 = case shown="True" w499 {
          tunnel: w528 -> [w622 w628]
          tunnel: [w622 w627] -> w527
          tunnel: w500 -> [_ w626]
          tunnel: w496 -> [_ w625]
          tunnel: w501 -> [_ w623]
          frame False {
          }
          frame True {
            n260 = call <vilib>:"DiffKinematics_New.vi"("TrackWidth_Meters"=w625) -> ("DIFF_DRIVE_KINEMATICS"=w624:T15)  [unwired: 10 in]
            n261 = call <vilib>:"TrajectoryConfig_setVoltageDiffDrive.vi"("SIMPLE_MOTOR_FF"=w626, "DIFF_DRIVE_KINEMATICS"=w624, "Max Voltage"=w623, "inTRAJECTORY_CONFIG"=w628) -> ("outTRAJECTORY_CONFIG"=w627:T29)  [unwired: 7 in]
          }
        }
        n262 = case shown="True" w502 {
          tunnel: [w575 w579] -> w519
          tunnel: w527 -> [w575 w578]
          tunnel: w503 -> [_ w576]
          frame False {
          }
          frame True {
            n263 = call <vilib>:"SwerveKinematics_NewX.vi"("Wheels"=w576) -> ("SWERVE_DRIVE_KINEMATICS"=w577:T18)  [unwired: 10 in]
            n264 = call <vilib>:"TrajectoryConfig_setKinematicsSwerveDrive.vi"("SWERVE_DRIVE_KINEMATICS"=w577, "inTRAJECTORY_CONFIG"=w578) -> ("outTRAJECTORY_CONFIG"=w579:T29)  [unwired: 9 in]
          }
        }
        n265 = case shown="True" w507 {
          tunnel: [w614 w621] -> w492
          tunnel: w519 -> [w614 w620]
          tunnel: w506 -> [_ w618]
          tunnel: w505 -> [_ w617]
          tunnel: w504 -> [_ w616]
          tunnel: w508 -> [_ w615]
          frame False {
          }
          frame True {
            n266 = call <vilib>:"MecaKinematics_New.vi"("RearRight"=w615, "RearLeft"=w616, "FrontRight"=w617, "FrontLeft"=w618) -> ("MECA_DRIVE_KINEMATICS"=w619:T23)  [unwired: 7 in]
            n267 = call <vilib>:"TrajectoryConfig_setKinematicsMecanumDrive.vi"("MECA_DRIVE_KINEMATICS"=w619, "inTRAJECTORY_CONFIG"=w620) -> ("outTRAJECTORY_CONFIG"=w621:T29)  [unwired: 9 in]
          }
        }
        n268 = case shown="\"Radio Selection 2\"" "Spline Type" {
          tunnel: [w591 w595] -> w516
          tunnel: w492 -> [w590 w593]
          tunnel: [w592 w596] -> w491
          tunnel: [TRUE FALSE] -> w490
          tunnel: w484 -> [w588 w598]
          tunnel: w479 -> [w582 w597]
          frame "Radio Selection 1", Default {
            # "format\nwaypoints for\nspline functions"
            # "Calc\ncubic\nsplines"
            n269 = call <vilib>:"Util_DispWeightedWaypoint_To_WeightedWayPoint.vi"("DisplayWeightedWayPoints"=w588) -> ("WeightedWayPoints"=w587:T35[])  [unwired: 10 in]
            n270 = call <vilib>:"SplineHelp_GetCubicCtrlVectorsFromWeightedWayPts.vi"("Use Weights"=w582, "WeightedWayPoints"=w587) -> ("Interior WAYPOINTS"=w586:T3[], "SplineControlVectors"=w585:T36[])  [unwired: 8 in]
            n271 = Index Array(array=w585, index #1=0 ("index"), index #2=1 ("index")) -> (element #1=w584:T36, element #2=w583:T36)
            n272 = call <vilib>:"TrajectoryGenerate_Make_Cubic_CtrlVect.vi"("traj_config"=w590, "end-Spline_Ctrl_Vector"=w583, "Interior WAYPOINTS"=w586, "initial-Spline_Ctrl_Vector"=w584) -> ("error out"=w591:errorcluster, "TRAJECTORY"=w592:T13)  [unwired: 6 in]
          }
          frame "Radio Selection 2" {
            # "format\nwaypoints for\nspline functions"
            # "CALC\nQUINTIC\nSPLINE"
            n273 = call <vilib>:"Util_DispWeightedWaypoint_To_WeightedWayPoint.vi"("DisplayWeightedWayPoints"=w598) -> ("WeightedWayPoints"=w594:T35[])  [unwired: 10 in]
            n274 = case shown="False" w597 {
              tunnel: [w604 w608] -> w596
              tunnel: [w603 w607] -> w595
              tunnel: w594 -> [w600 w606]
              tunnel: w593 -> [w601 w605]
              frame False {
                n275 = call "Create_Trajectory_Weighted_to_NonWeighted.vi"("WeightedWayPoints"=w600) -> ("WayPoints"=w602:T8[])  [unwired: 10 in]
                n276 = call <vilib>:"TrajectoryGenerate_Make_Quintic.vi"("traj_config"=w601, "waypointPOSE"=w602) -> ("error out"=w603:errorcluster, "TRAJECTORY"=w604:T13)  [unwired: 8 in]
              }
              frame True {
                n277 = call <vilib>:"TrajectoryGenerate_Make_Quintic_Weighted.vi"("traj_config"=w605, "WeightedWaypointPOSE"=w606) -> ("error out"=w607:errorcluster, "TRAJECTORY"=w608:T13)  [unwired: 8 in]
              }
            }
          }
        }
        "Trajectory calculation error" <- w516
        n278 = Unbundle By Name(w491) -> ("States"=w522:T7[], "TotalTImeSecs"=w526:dbl)
        "Trajectory States" <- w522
        n279 = while {
          tunnel: [w567] -> w464 mode=indexing
          tunnel: [w558] -> w474 mode=indexing
          tunnel: [w560] -> w473 mode=indexing
          tunnel: [w564] -> w472 mode=indexing
          tunnel: [w559] -> w471 mode=indexing
          tunnel: [w574] -> w470 mode=indexing
          shift-right: [w568] -> _
          shift-left: 0.0 -> [w558]
          tunnel: [w562] -> w463 mode=indexing
          tunnel: w526 -> [w554]
          tunnel: w491 -> [w546]
          i -> [w552]
          stop <- w553 stop-if-true
          # "Time Df"
          # "Jerk"
          # "Dist"
          n280 = To Double Precision Float(number=w552) -> (double precision float=w551:dbl)
          n281 = Multiply(x=w551, y=0.02) -> (x*y=w549:dbl)
          n282 = feedback #14(0.0 ("TimeSeconds")) -> (w570:dbl)
          n283 = feedback #15(0.0 ("TimeSeconds")) -> (w572:dbl)
          n284 = feedback #16(0.0 ("TimeSeconds")) -> (w565:dbl)
          n285 = call <vilib>:"Trajectory_Sample.vi"("Time"=w549, "InputTRAJECTORY"=w546) -> ("OutputTRAJ_STATE"=w547:T7)  [unwired: 9 in]
          n286 = call <vilib>:"Util_TrajectoryState_Meters_To_Inches.vi"("absTRAJECTORY"=w547) -> ("outputRelativeTRAJECTORY"=w548:T7)  [unwired: 10 in]
          n287 = Unbundle By Name(w548) -> ("TimeSeconds"=w567:dbl, "Velocity"=w560:dbl, "Acceleration"=w564:dbl, "Curvature"=w561:dbl, "POSE.ROTATION.VALUE"=w574:dbl)
          n288 = feedback-in #14(w560) -> ()
          n289 = feedback-in #15(w567) -> ()
          n290 = feedback-in #16(w564) -> ()
          n291 = Add(x=w560, y=w570) -> (x+y=w569:dbl)
          n292 = Subtract(x=w567, y=w572) -> (x-y=w555:dbl)
          n293 = Subtract(x=w564, y=w565) -> (x-y=w563:dbl)
          n294 = Compound Arithmetic op=MULTIPLY(w569, 0.5 ("value"), w555) -> (w557:dbl)
          n295 = Divide(x=w563, y=w555) -> (x/y=w562:dbl)
          n296 = Add(x=w557, y=w558) -> (x+y=w568:dbl)
          n297 = Greater Or Equal?(x=w549, y=w554) -> (x >= y?=w553:bool)
          n298 = Multiply(x=w560, y=w561) -> (x*y=w559:dbl)
        }
        n299 = for {
          tunnel: w522 -> [w633] mode=indexing
          tunnel: w496 -> [w642]
          tunnel: [w640] -> w535 mode=indexing
          tunnel: [w639] -> w534 mode=indexing
          tunnel: [w636] -> w533 mode=indexing
          tunnel: [w634] -> w532 mode=indexing
          tunnel: [w630] -> w525 mode=indexing
          tunnel: [w629] -> w524 mode=indexing
          n300 = Unbundle By Name(w633) -> ("POSE.TRANSLATION.X"=w632:dbl, "POSE.TRANSLATION.Y"=w631:dbl)
          n301 = call <vilib>:"Util_TrajState_to_DiffDrive_WheelPos.vi"("Wheelbase"=w642, "TRAJ_STATE"=w633) -> ("Right Y"=w635:dbl, "Right X"=w637:dbl, "Left Y"=w638:dbl, "Left X"=w641:dbl)  [unwired: 6 in]
          n302 = call <vilib>:"Conv_Meters_Inches.vi"("Meters"=w641) -> ("Inches"=w640:dbl)  [unwired: 10 in]
          n303 = call <vilib>:"Conv_Meters_Inches.vi"("Meters"=w637) -> ("Inches"=w636:dbl)  [unwired: 10 in]
          n304 = call <vilib>:"Conv_Meters_Inches.vi"("Meters"=w632) -> ("Inches"=w629:dbl)  [unwired: 10 in]
          n305 = call <vilib>:"Conv_Meters_Inches.vi"("Meters"=w638) -> ("Inches"=w639:dbl)  [unwired: 10 in]
          n306 = call <vilib>:"Conv_Meters_Inches.vi"("Meters"=w635) -> ("Inches"=w634:dbl)  [unwired: 10 in]
          n307 = call <vilib>:"Conv_Meters_Inches.vi"("Meters"=w631) -> ("Inches"=w630:dbl)  [unwired: 10 in]
        }
        n308 = for {
          tunnel: [w652] -> w543 mode=indexing
          tunnel: [w651] -> w541 mode=indexing
          tunnel: w522 -> [w659] mode=indexing
          tunnel: w523 -> [w653]
          # "see if max speed violated  by\neither wheel speed"
          n309 = Unbundle By Name(w659) -> ("Velocity"=w657:dbl, "Curvature"=w658:dbl)
          n310 = Multiply(x=w657, y=w658) -> (x*y=w655:dbl)
          n311 = call <vilib>:"ChassisSpeeds_New.vi"("vAngular"=w655, "vY"=0.0, "vX"=w657) -> ("CHASSIS"=w654:T37)  [unwired: 8 in]
          n312 = call <vilib>:"DiffKinematics_toWheelSpeed.vi"("CHASSIS Speed"=w654, "DIFF_DRIVE_KINEMATICS"=w653) -> ("RightVelocity"=w651:dbl, "LeftVelocity"=w652:dbl)  [unwired: 8 in]
        }
        n313 = Bundle(w483, w482) -> (w481:cluster{dbl[], dbl[]})  [unwired: 1 in]
        n314 = Bundle(w524, w525) -> (w530:cluster{dbl[], dbl[]})  [unwired: 1 in]
        n315 = Bundle(w535, w534) -> (w529:cluster{dbl[], dbl[]})  [unwired: 1 in]
        n316 = Bundle(w533, w532) -> (w531:cluster{dbl[], dbl[]})  [unwired: 1 in]
        n317 = Absolute Value(x=w543) -> (abs(x)=w542:dbl[])
        n318 = Absolute Value(x=w541) -> (abs(x)=w540:dbl[])
        n319 = Multiply(x=w493, y=1.01) -> (x*y=w517:dbl)
        n320 = Build Array(w530, w529, w531, w481) -> (→"Position":cluster{dbl[], dbl[]}[])
        n321 = Array Max & Min(array=w542) -> (max value=w538:dbl)  [unwired: 3 out]
        n322 = Array Max & Min(array=w540) -> (max value=w537:dbl)  [unwired: 3 out]
        n323 = Greater?(x=w538, y=w517) -> (0:w544:bool)
        n324 = Greater?(x=w537, y=w517) -> (0:w539:bool)
        n325 = Max & Min(x=w538, y=w537) -> (max(x,y)=w521:dbl)  [unwired: 1 out]
        n326 = Bundle(w464, w471) -> (w469:cluster{dbl[], dbl[]})  [unwired: 1 in]
        n327 = Bundle(w464, w470) -> (w468:cluster{dbl[], dbl[]})  [unwired: 1 in]
        n328 = Bundle(w464, w473) -> (w476:cluster{dbl[], dbl[]})  [unwired: 1 in]
        n329 = Bundle(w464, w463) -> (w465:cluster{dbl[], dbl[]})  [unwired: 1 in]
        n330 = Bundle(w464, w474) -> (w477:cluster{dbl[], dbl[]})  [unwired: 1 in]
        n331 = Bundle(w464, w472) -> (w475:cluster{dbl[], dbl[]})  [unwired: 1 in]
        n332 = Compound Arithmetic op=OR(w544, w539) -> (w488:bool)
        n333 = call <vilib>:"Conv_Meters_Inches.vi"("Meters"=w521) -> ("Inches"=→"differential \ndrive \nmax speed":dbl)  [unwired: 10 in]
        n334 = Array Size(array=w522) -> (size(s)=w514:i32)
        "Traj States\nSize" <- w514
        n335 = Build Array(w477, w476, w475, w469, w468, w465) -> (→"Trajectory Data":cluster{dbl[], dbl[]}[])
        n336 = And(x=w488, y=w487) -> (x .and. y?=w486:bool)
        n337 = Not(x=w486) -> (.not. x?=w512:bool)
        n338 = Greater Than 0?(x=w514) -> (x > 0?=w513:bool)
        n339 = And(x=w513, y=w512) -> (x .and. y?=w515:bool)
      }
      frame 3 {
        # "Write trajectory to CSV File"
        n340 = case shown="\"Radio Selection 1\", Default" w661 {
          tunnel: w689 -> [w699 w701]
          tunnel: [w698 w701] -> w693
          tunnel: [TRUE FALSE] -> w691
          frame "Radio Selection 1", Default {
            # "Relative"
            n341 = call <vilib>:"Util_Trajectory_Absolute_To_Relative.vi"("absTRAJECTORY"=w699) -> ("outputRelativeTRAJECTORY"=w698:T13)  [unwired: 10 in]
          }
          frame "Radio Selection 2" {
            # "Absolute"
          }
        }
        n342 = call <vilib>:"Util_Trajectory_WriteFile.vi"("Trajectory is Cubic"=w687, "UseWeights"=w663, "Trajectory Is Relative"=w691, "TRAJECTORY_CONFIG"=w688, "UtilityWayPoints"=w664, "TRAJECTORY"=w693, "Comment"="Trajectory File Comment", "Trajectory File Name"="Trajectory CSV File Name") -> ("error out"=w692:errorcluster)  [unwired: 3 in]
        "Write Trajectory\nFile Error" <- w692
        n343 = local write "Write Config File Comment"("Trajectory File Comment") -> ()
        n344 = case shown="Error .." w692 {
          tunnel: [TRUE ("File Saved\nWithout\nError") FALSE ("File Saved\nWithout\nError")] -> w685
          frame No Error {
          }
          frame Error {
          }
        }
      }
      frame 4 {
        # "Write trajectory to JSON File"
        n345 = case shown="\"Radio Selection 1\", Default" w711 {
          tunnel: w738 -> [w838 w840]
          tunnel: [w837 w840] -> w707
          tunnel: [TRUE FALSE] -> _
          frame "Radio Selection 1", Default {
            # "Relative"
            n346 = call <vilib>:"Util_Trajectory_Absolute_To_Relative.vi"("absTRAJECTORY"=w838) -> ("outputRelativeTRAJECTORY"=w837:T13)  [unwired: 10 in]
          }
          frame "Radio Selection 2" {
            # "Absolute"
          }
        }
        n347 = Unbundle By Name(w707) -> ("States"=w706:T7[])
        n348 = case shown="\"Radio Selection 1\"" "PathWeaver Length Units" {
          tunnel: w706 -> [w740 w741 w765 w795 w815]
          tunnel: [w740 w742 w764 w794 w814] -> w703
          frame "Radio Selection 1" {
            # "Meters - do nothing"
          }
          frame "Radio Selection 2" {
            # "Conv Meters to Centimeters"
            n349 = for {
              tunnel: w741 -> [w744] mode=indexing
              tunnel: [w743] -> w742 mode=indexing
              n350 = in-place {
                n351 = in-place-cluster #17(w744) -> ("Acceleration"=w755:dbl, "TimeSeconds"=w763:dbl, "Velocity"=w753:dbl, "Curvature"=w758:dbl, "POSE.TRANSLATION.X"=w745:dbl, "POSE.TRANSLATION.Y"=w749:dbl, "POSE.ROTATION.VALUE"=w760:dbl, "POSE.ROTATION.COS"=w762:dbl, "POSE.ROTATION.SIN"=w761:dbl)
                n352 = Multiply(x=w745, y=100.0) -> (x*y=w746:dbl)
                n353 = Multiply(x=w749, y=100.0) -> (x*y=w748:dbl)
                n354 = Multiply(x=w753, y=100.0) -> (x*y=w752:dbl)
                n355 = Multiply(x=w755, y=100.0) -> (x*y=w756:dbl)
                n356 = Divide(x=w758, y=100.0 ("Centimeter")) -> (x/y=w759:dbl)
                n357 = in-place-cluster #17("Acceleration"=w756, "TimeSeconds"=w763, "Velocity"=w752, "Curvature"=w759, "POSE.TRANSLATION.X"=w746, "POSE.TRANSLATION.Y"=w748, "POSE.ROTATION.VALUE"=w760, "POSE.ROTATION.COS"=w762, "POSE.ROTATION.SIN"=w761) -> (w743:T7)
              }
            }
          }
          frame "Radio Selection 3" {
            # "Who uses yards ????"
            # "Conv Meters to Yards"
            n358 = for {
              tunnel: w765 -> [w767] mode=indexing
              tunnel: [w766] -> w764 mode=indexing
              n359 = in-place {
                n360 = in-place-cluster #18(w767) -> ("Acceleration"=w787:dbl, "TimeSeconds"=w793:dbl, "Velocity"=w788:dbl, "Curvature"=w785:dbl, "POSE.TRANSLATION.X"=w789:dbl, "POSE.TRANSLATION.Y"=w790:dbl, "POSE.ROTATION.VALUE"=w786:dbl, "POSE.ROTATION.COS"=w792:dbl, "POSE.ROTATION.SIN"=w791:dbl)
                n361 = call <vilib>:"Conv_Meters_Feet.vi"("Meters"=w790) -> ("Feet"=w772:dbl)  [unwired: 10 in]
                n362 = call <vilib>:"Conv_Meters_Feet.vi"("Meters"=w787) -> ("Feet"=w782:dbl)  [unwired: 10 in]
                n363 = call <vilib>:"Conv_Meters_Feet.vi"("Meters"=w788) -> ("Feet"=w778:dbl)  [unwired: 10 in]
                n364 = call <vilib>:"Conv_Meters_Feet.vi"("Meters"=w789) -> ("Feet"=w769:dbl)  [unwired: 10 in]
                n365 = Divide(x=w769, y=3.0) -> (x/y=w768:dbl)
                n366 = Divide(x=w772, y=3.0) -> (x/y=w771:dbl)
                n367 = Divide(x=w782, y=3.0) -> (x/y=w780:dbl)
                n368 = Divide(x=w778, y=3.0) -> (x/y=w777:dbl)
                n369 = call <vilib>:"Conv_Meters_Feet.vi"("Meters"=1.0 ("Centimeter")) -> ("Feet"=w774:dbl)  [unwired: 10 in]
                n370 = Divide(x=w774, y=3.0) -> (x/y=w775:dbl)
                n371 = Divide(x=w785, y=w775) -> (x/y=w784:dbl)
                n372 = in-place-cluster #18("Acceleration"=w780, "TimeSeconds"=w793, "Velocity"=w777, "Curvature"=w784, "POSE.TRANSLATION.X"=w768, "POSE.TRANSLATION.Y"=w771, "POSE.ROTATION.VALUE"=w786, "POSE.ROTATION.COS"=w792, "POSE.ROTATION.SIN"=w791) -> (w766:T7)
              }
            }
          }
          frame "Radio Selection 4" {
            # "Meters Conv to Feet"
            n373 = for {
              tunnel: w795 -> [w797] mode=indexing
              tunnel: [w796] -> w794 mode=indexing
              n374 = in-place {
                n375 = in-place-cluster #19(w797) -> ("Acceleration"=w805:dbl, "TimeSeconds"=w813:dbl, "Velocity"=w807:dbl, "Curvature"=w799:dbl, "POSE.TRANSLATION.X"=w809:dbl, "POSE.TRANSLATION.Y"=w810:dbl, "POSE.ROTATION.VALUE"=w802:dbl, "POSE.ROTATION.COS"=w812:dbl, "POSE.ROTATION.SIN"=w811:dbl)
                n376 = call <vilib>:"Conv_Meters_Feet.vi"("Meters"=w805) -> ("Feet"=w804:dbl)  [unwired: 10 in]
                n377 = call <vilib>:"Conv_Meters_Feet.vi"("Meters"=w807) -> ("Feet"=w806:dbl)  [unwired: 10 in]
                n378 = call <vilib>:"Conv_Meters_Feet.vi"("Meters"=w809) -> ("Feet"=w808:dbl)  [unwired: 10 in]
                n379 = call <vilib>:"Conv_Meters_Feet.vi"("Meters"=w810) -> ("Feet"=w803:dbl)  [unwired: 10 in]
                n380 = call <vilib>:"Conv_Meters_Feet.vi"("Meters"=1.0 ("Centimeter")) -> ("Feet"=w800:dbl)  [unwired: 10 in]
                n381 = Divide(x=w799, y=w800) -> (x/y=w798:dbl)
                n382 = in-place-cluster #19("Acceleration"=w804, "TimeSeconds"=w813, "Velocity"=w806, "Curvature"=w798, "POSE.TRANSLATION.X"=w808, "POSE.TRANSLATION.Y"=w803, "POSE.ROTATION.VALUE"=w802, "POSE.ROTATION.COS"=w812, "POSE.ROTATION.SIN"=w811) -> (w796:T7)
              }
            }
          }
          frame "Radio Selection 5" {
            # "Meters - Conv to Inches"
            n383 = for {
              tunnel: w815 -> [w817] mode=indexing
              tunnel: [w816] -> w814 mode=indexing
              n384 = in-place {
                n385 = in-place-cluster #20(w817) -> ("Acceleration"=w825:dbl, "TimeSeconds"=w833:dbl, "Velocity"=w827:dbl, "Curvature"=w819:dbl, "POSE.TRANSLATION.X"=w829:dbl, "POSE.TRANSLATION.Y"=w830:dbl, "POSE.ROTATION.VALUE"=w822:dbl, "POSE.ROTATION.COS"=w832:dbl, "POSE.ROTATION.SIN"=w831:dbl)
                n386 = call <vilib>:"Conv_Meters_Inches.vi"("Meters"=w825) -> ("Inches"=w824:dbl)  [unwired: 10 in]
                n387 = call <vilib>:"Conv_Meters_Inches.vi"("Meters"=w827) -> ("Inches"=w826:dbl)  [unwired: 10 in]
                n388 = call <vilib>:"Conv_Meters_Inches.vi"("Meters"=w829) -> ("Inches"=w828:dbl)  [unwired: 10 in]
                n389 = call <vilib>:"Conv_Meters_Inches.vi"("Meters"=w830) -> ("Inches"=w823:dbl)  [unwired: 10 in]
                n390 = call <vilib>:"Conv_Meters_Inches.vi"("Meters"=1.0 ("Centimeter")) -> ("Inches"=w820:dbl)  [unwired: 10 in]
                n391 = Divide(x=w819, y=w820) -> (x/y=w818:dbl)
                n392 = in-place-cluster #20("Acceleration"=w824, "TimeSeconds"=w833, "Velocity"=w826, "Curvature"=w818, "POSE.TRANSLATION.X"=w828, "POSE.TRANSLATION.Y"=w823, "POSE.ROTATION.VALUE"=w822, "POSE.ROTATION.COS"=w832, "POSE.ROTATION.SIN"=w831) -> (w816:T7)
              }
            }
          }
        }
        n393 = call <vilib>:"Trajectory_New.vi"("TRAJ_STATES"=w703) -> ("TRAJECTORY"=w704:T13)  [unwired: 10 in]
        n394 = Path To String(path="Trajectory JSON File Name") -> (string=w709:string)
        n395 = call <vilib>:"TrajectoryUtil_toPathWeaverJSON.vi"("inTRAJECTORY"=w704, "FileName"=w709) -> ("error out"=w710:errorcluster)  [unwired: 8 in, 1 out]
        "Write CSV File Error" <- w710
        n396 = case shown="Error .." w710 {
          tunnel: [TRUE ("File Saved\nWithout\nError") FALSE ("File Saved\nWithout\nError")] -> w713
          frame No Error {
          }
          frame Error {
          }
        }
      }
      frame 5 {
        # "write xml\nfile"
        # "convert\nto xml\nstring"
        # "Write config to File"
        n397 = Bundle By Name(cluster=T14 {"Write Config File Name"=path "", "Write Config File Comment"="", "WayPoints"=[], "TRAJECTORY_CONFIG"={"MaxVelocity"=0.0, "Max Acceleration"=0.0, "StartVelocity"=0.0, "End Velocity"=0.0, "Reversed"=FALSE, "DiffDrKineConstntDefined"=FALSE, "CentAcellConstntDefined"=FALSE, "DiffDrVoltConstntDefined"=FALSE, "DIFF_DRIVE_KINE_CONSTRAINT"={"Max Speed (M/S)"=0.0, "DIFF_DRIVE_KINEMATICS"={"TrackWidth_Meters"=0.0}}, "CENTRIPETAL_ACCEL_CONSTRAINT"={"Max Cent Accel"=0.0}, "SwerveDrKineConstntDefined"=FALSE, "SWERVE_DRIVE_KINE_CONSTRAINT"={"Max Speed (M/S)"=0.0, "SwerveKinematics"={"NumModules"=0, "InverseKinematics"=[], "ForwardKinematics"=[], "Modules"=[], "PrevCoR"={"X"=0.0, "Y"=0.0}, "SavedModuleStates"=[]}}, "DIFF_DRIVE_VOLTAGE_CONSTRAINT"={"Max Voltage"=0.0, "DIFF_DRIVE_KINEMATICS"={"TrackWidth_Meters"=0.0}, "SIMPLE_MOTOR_FF"={"Ks"=0.0, "Kv"=0.0, "Ka"=0.0, "KnInv"=0.0}}, "MECANUM_DRIVE_KINE_CONSTRAINT"={"Max Speed (M/S)"=0.0, "MECA_DRIVE_KINEMATICS"={"FrontLeft"={"X"=0.0, "Y"=0.0}, "FrontRight"={"X"=0.0, "Y"=0.0}, "RearLeft"={"X"=0.0, "Y"=0.0}, "RearRight"={"X"=0.0, "Y"=0.0}, "InverseKinematics"=[], "ForwardKinematics"=[], "PrevCoR"={"X"=0.0, "Y"=0.0}}}, "MecanumDrKineConstntDefined"=FALSE}, "IsCubic"=FALSE, "Units Selector"=enum."Inches", "UseWeights"=FALSE} ("TrajCreateConfig"), "Write Config File Name"="Write Config File Name", "Write Config File Comment"="Write Config File Comment", "WayPoints"=w856, "TRAJECTORY_CONFIG"=w855, "IsCubic"=w854, "Units Selector"=w845, "UseWeights"=w843) -> (w852:T14)
        n398 = local write "Trajectory File Comment"("Write Config File Comment") -> ()
        n399 = Flatten To XML(anything=w852) -> (xml string=w850:string)
        n400 = call-poly <vilib>:"Write to XML File.vi"("Standalone? (T)"=TRUE, "XML Input"=w850, "XML File Path"="Write Config File Name") -> ("error out"=w848:errorcluster)  [unwired: 6 in, 2 out]
        "Write Config FIle Error" <- w848
        n401 = case shown="No Error" w848 {
          tunnel: [TRUE ("File Saved\nWithout\nError") FALSE ("File Saved\nWithout\nError")] -> w847
          frame No Error {
          }
          frame Error {
          }
        }
      }
      frame 6 {
        # "End Program"
        n402 = disable-structure shown="Default" {
          frame condition #0 (active) {
            n403 = Stop() -> ()  [unwired: 1 in]
          }
          frame condition #1 {
            n404 = Quit LabVIEW() -> ()  [unwired: 1 in]
          }
        }
      }
    }
    "Trajectory\nCompleted\nError Free" <- w110
    "CSV File Saved\nWithout Error" <- w106
    "Config File Saved\nWithout Error" <- w60
    "JSON File Saved\nWithout Error" <- w45
  }
  "Index" <- 0 ("index")
